vi "SynthApp.vi"(0 "Choose Directory":path, 1 "Show SF?":bool=TRUE, 2 "Show Sum?":bool, 3 "Save Center\nElem?":bool, 5 "Auto Select All?":bool, 7 "Use Selected Files":bool, 9 "Trans Geometry (mm)":T1={"Transducer"=0, "Geo Focus"=12.0, "a (radius)"=3.0, "# of rings"=5, "kerf space "=0.1, "Center Freq"=12.0} {"Transducer" items=["6D 12R 40 MHz"=0, "10D 31R 20 MHz"=1, "10D 23R 20 MHz"=2, "6D 23R 40 MHz"=3, "4.5D 10.7R 40 MHz"=4, "9D 23.5R 20 MHz"=5, "9D 25.8R 20MHz"=6, "Enter"=99]}, 11 "Method":u16(ring)=4 items=["Normal", "GPU", "ABUT", "EXPAND", "CPU"], 12 "Save Data":bool, 13 "Type of Mean":T3=enum."Filter", 14 "Filter Prams":T4={"low cutoff"=5, "order"=51, "high cutoff"=65}) -> ()   [LabVIEW 2022 SP3]
uses:
  ViewData/-ReadEye/TypeDefs/TypeofMean.ctl
  -AnnularRoutines/TransGeometry.ctl
  -AnnularRoutines/ArrayGeometry.ctl
  -AnnularRoutines/AnnularArray.ctl
  <vilib>/Analysis/4window.llb/Chebyshev Window (DBL).vi
  -SynthApperture/FastArraySum.vi
  -SynthApperture/FastArraySumSGL.vi
  <vilib>/Analysis/NI_AALBase.lvlib
  <vilib>/Analysis/NI_AALPro.lvlib
  GPU_HK/LabVIEW Example/riversideSAFilter-X64.dll
panel:
  in  "offset dual (mm)":dbl=15.0
  in  "Special Two Way":bool
  in  "Nested Files?":bool
  in  "Save Tiff?":bool
  in  "index (row)":i32
  out "Waveform Graph":dbl[][](graph)
  in  "downfactor":i32=1
  in  "Xmt/Rcv":cluster{"XMIT":bool[], "RCV":bool[]}={"XMIT"=[TRUE, TRUE, TRUE, TRUE, TRUE], "RCV"=[TRUE, TRUE, TRUE, TRUE, TRUE]}
  out "Comment":string
  out "Recip Table":i16[][](array[numeric])
  in  "delay":sgl format="%_3f"
  out "annuli rad (mm)":dbl[](array[numeric])
  in  "Special Save":bool
  out "GPU time (ms)":u32
  out "nError":i32
  in  "Scale Voltage?":bool=TRUE
  out "time per\nimage (ms)":u32
  in  "One Way Receive":bool
  in  "Compression Parameters.% taper":sgl
  in  "Display Plots":bool=TRUE
  in  "Axis scaling":bool=TRUE
  in  "Compress":bool
  in  "Round to ROC?":bool=TRUE
  out "ROC (m)":dbl=0.012
  out "Current File":string
  in  "file ext":string="*1to1*"
  out "zone size mm":dbl format="%#_3g"
  in  "Normalize Voltages":bool
  in  "c (m/s)":i32=1485
  out "Raw Summation":dbl[][](graph)
  in  "F- zones":i16=41
  out "Focal zones m":sgl[](array[numeric])=[0.0085, 0.009, 0.0095, 0.01, 0.0105, 0.011, 0.0115, 0.012, 0.0125, 0.013, 0.0135, 0.014, 0.0145, 0.015]
  out "Synth Aperture":dbl[][](graph)
  in  "Listbox":i32[](listbox)
  # "Dynamic Receive"
  # "RCV"
  # "XMIT"
  # "Obsolete"
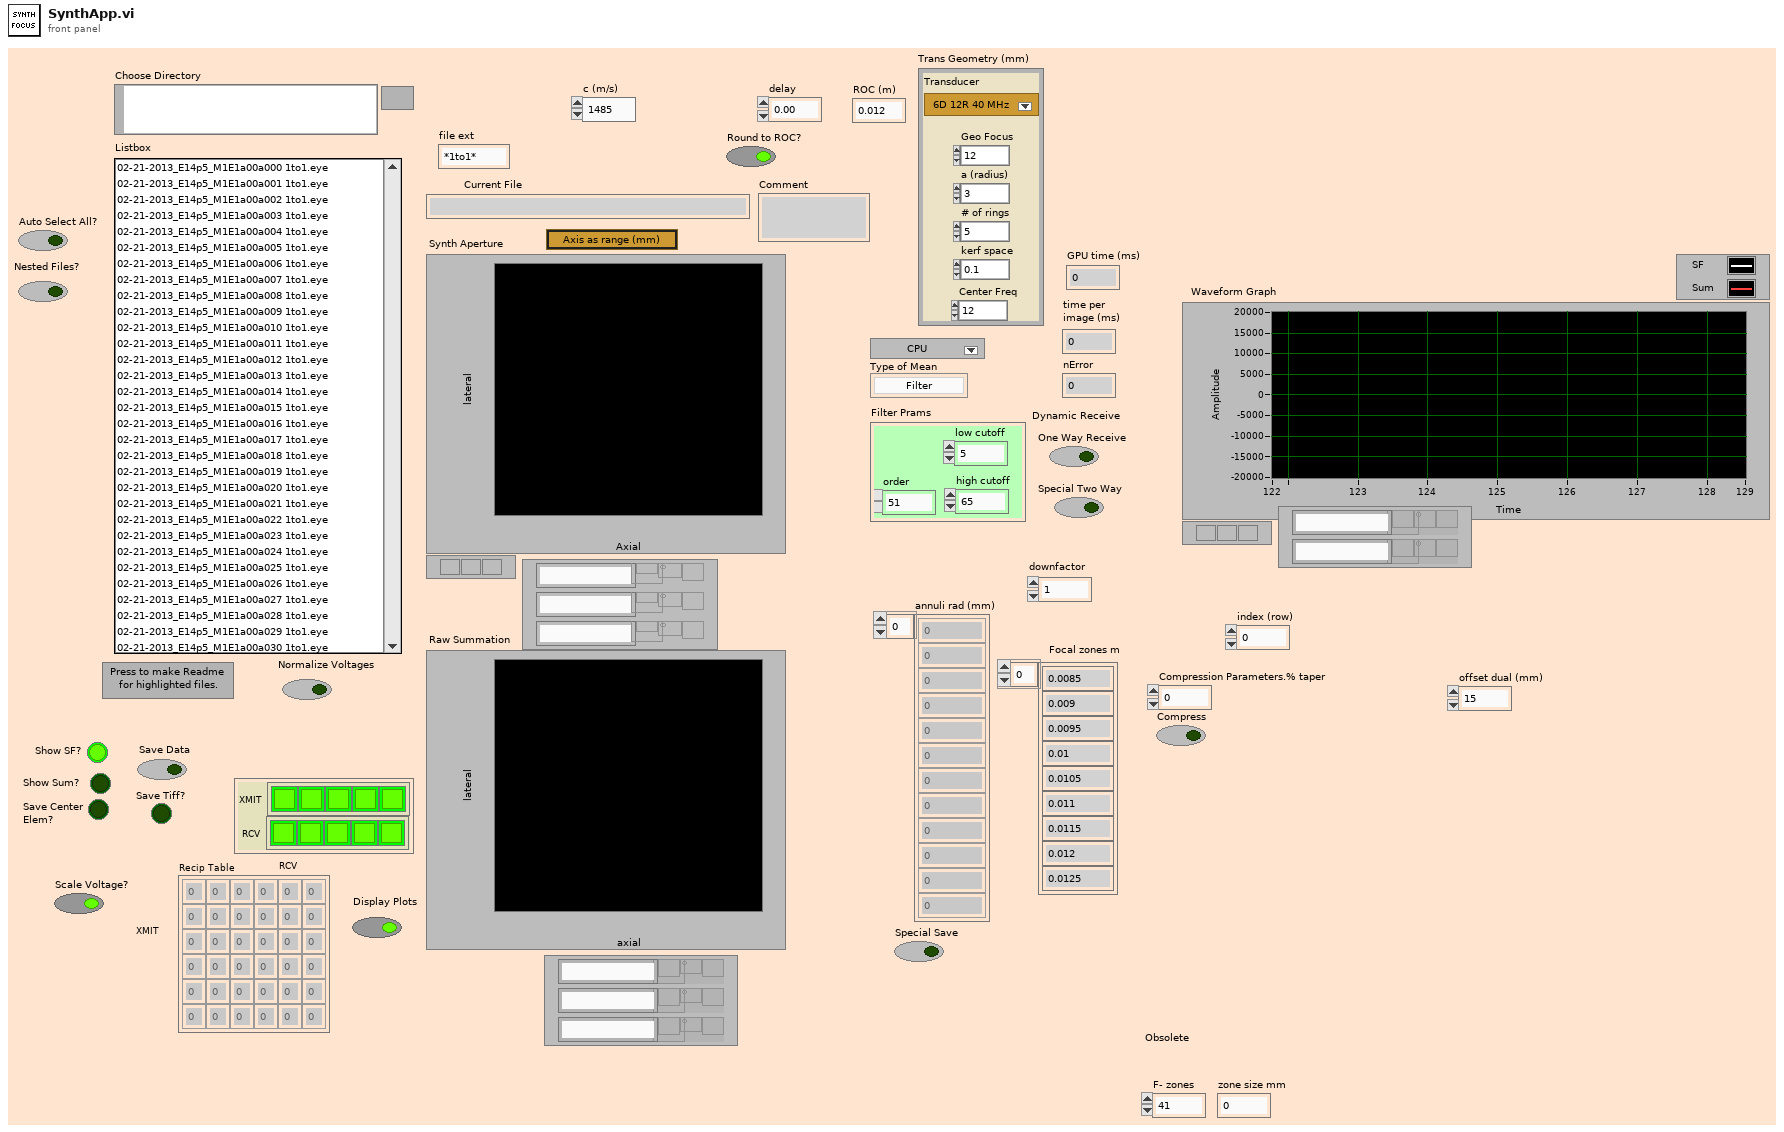
[diagram p1: front panel]
types:
  T1 = typedef "TransGeometry.ctl" = cluster{"Transducer":T2, "Geo Focus":dbl, "a (radius)":dbl, "# of rings":i32, "kerf space ":dbl, "Center Freq":dbl}
  T2 = typedef "ArrayGeometry.ctl" = u16
  T3 = typedef "TypeofMean.ctl" = enum16{"Mean from lines", "Mean just lines", "Poly Mean", "No mean", "Filter"}
  T4 = cluster{"low cutoff":i32, "order":i32, "high cutoff":i32}
  T5 = typedef "AnnularArray.ctl" = cluster{"Synth Foc?":bool, "Focal Zones":i16, "Switch T/R":i16, "Trans Geometry (mm)":T1, "Sub Ap Excite?":bool, "Full Array Scan?":bool, "Xmt/Rcv":cluster{"XMIT":bool[], "RCV":bool[]}, "PulseSpacing (us)":sgl, "Xmit Ring":i32, "XMIT CHS":u8, "RCV CHS":u8, "GPU?":bool, "Save TIFF?":bool, "downfactor":i32, "RCV 1CH":u16}
  T6 = cluster{"txPos":i32[], "rxPos":i32[], "Weights":i16[], "Ones":i16[]}
  T7 = typedef "Header.ctl" = cluster{"header info":cluster{"Header":string, "Head length":i16}, "A/D info":cluster{"# rf points per line":u16, "# lines per scan":u16, "sample rate MHz":u16, "# A/D bits":i16, "# bytes per A/D":u16, "TGC Flag":u16, "A/D Type":string}, "Tranducer Info":cluster{"bandwidth":sgl, "center freq":sgl, "start freq":sgl, "ID":i32}, "Scan Info":cluster{"delay":sgl, "pivot distance":sgl, "sector scan angle":sgl, "operator":string, "Scan Mode":string, "location":string}, "Time/Date Info":cluster{"date":string, "time":string}, "RF Info":cluster{"RF file name":string, "RF file att":string, "RF cal file name":string, "RF cal file att":string}, "Patient Info":cluster{"ID":string, "extended ID":string, "age":u16, "sex":string, "previously\nscanned":string, "PSA":sgl, "LOS":u8, "Ethnicty 2":u8, "Race":u8}, "Tissue Type":cluster{"organ":i16, "disease type":i16, "disease location":i16, "IQ_pts":u16, "RcvBuffer":u8, "RcvFrame":u16, "IQBuff":u8, "IQFrame":u16, "IQPage":u8}, "Votage scaling":cluster{"Digitizer (dB)":sgl, "Gain (dB)":sgl, "Atten (dB)":sgl}, "Comment":string, "Misc Info":cluster{"avg num":u16, "c speed":i16, "Div By or SF zones":i16, "XMIT CHS":u8, "RCV CHS":u8, "Xmit angle":sgl}, "Therapy Parameters":cluster{"Theraputic Freq (MHz)":sgl, "Time on (s)":sgl, "Therapy amplitude (mV)":sgl, "Lines Before":u16, "Lines After":u16}, "Scan Settings":cluster{"Energy (uJ or V)":u8, "Damp (Ohm) or Fc":u8, "HP Filt (KHz)":u8, "LP Filt (MHz)":u8, "Gain (db)":u8, "prf (kHz)":sgl, "Distance between\nscan lines (um)":u16, "Distance between\nscan planes (um)":u16, "Scan line gap (um)":sgl, "Scan plane gap (um)":sgl}, "Compression Parameters":cluster{"F1 (MHz)":sgl, "F2 (MHz)":sgl, "% taper":sgl, "duration":sgl}, "Patient Info Xtra":cluster{"First Name":string, "Last Name":string, "Notes":string}, "ROI Box":u16[]}
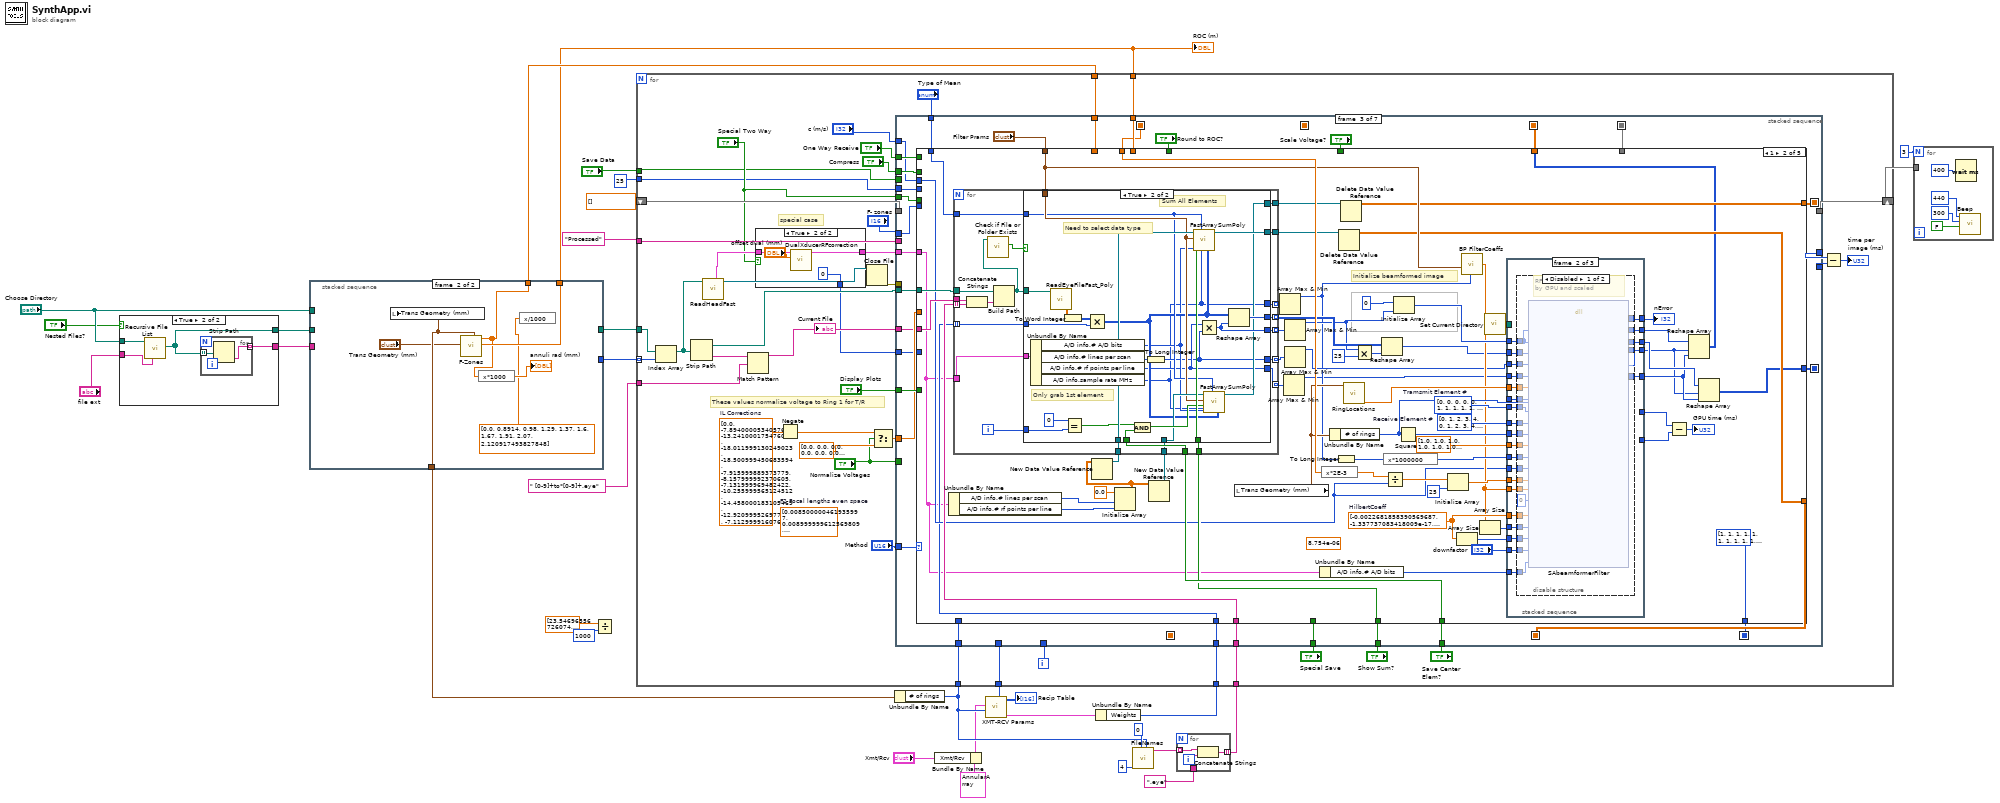
[diagram p0: block diagram]
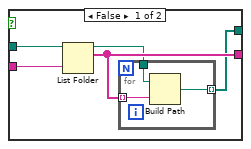
[diagram p2: hidden frame]
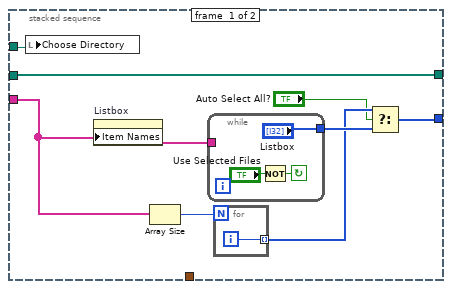
[diagram p3: hidden frame]
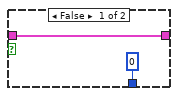
[diagram p4: hidden frame]
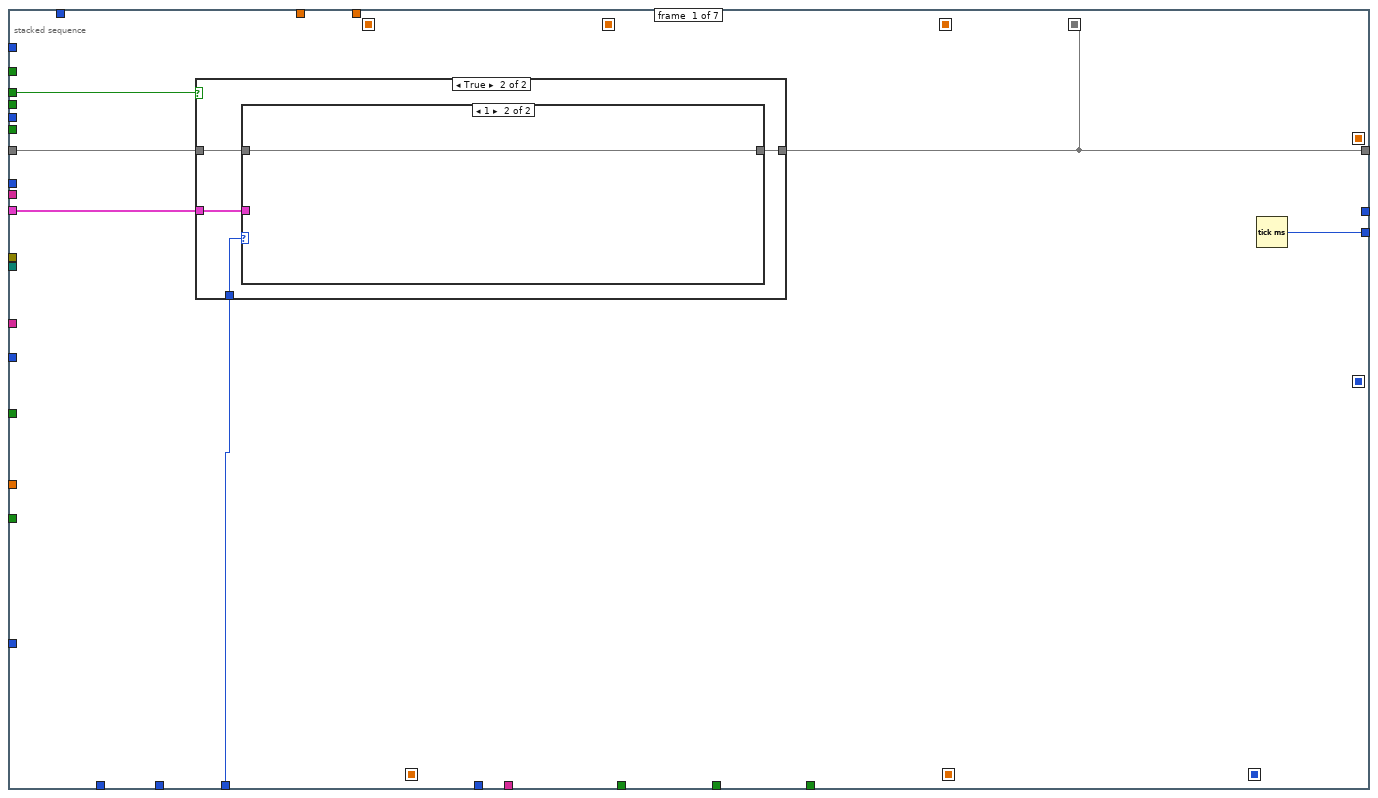
[diagram p5: hidden frame]
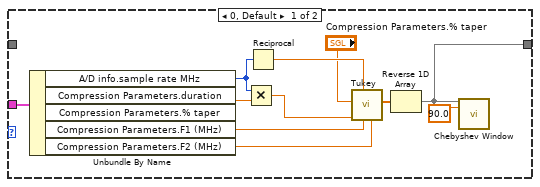
[diagram p7: hidden frame]
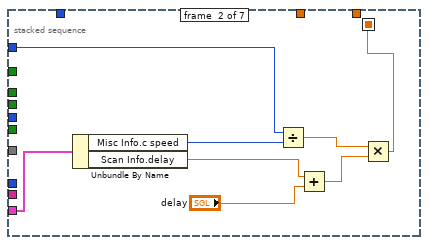
[diagram p8: hidden frame]
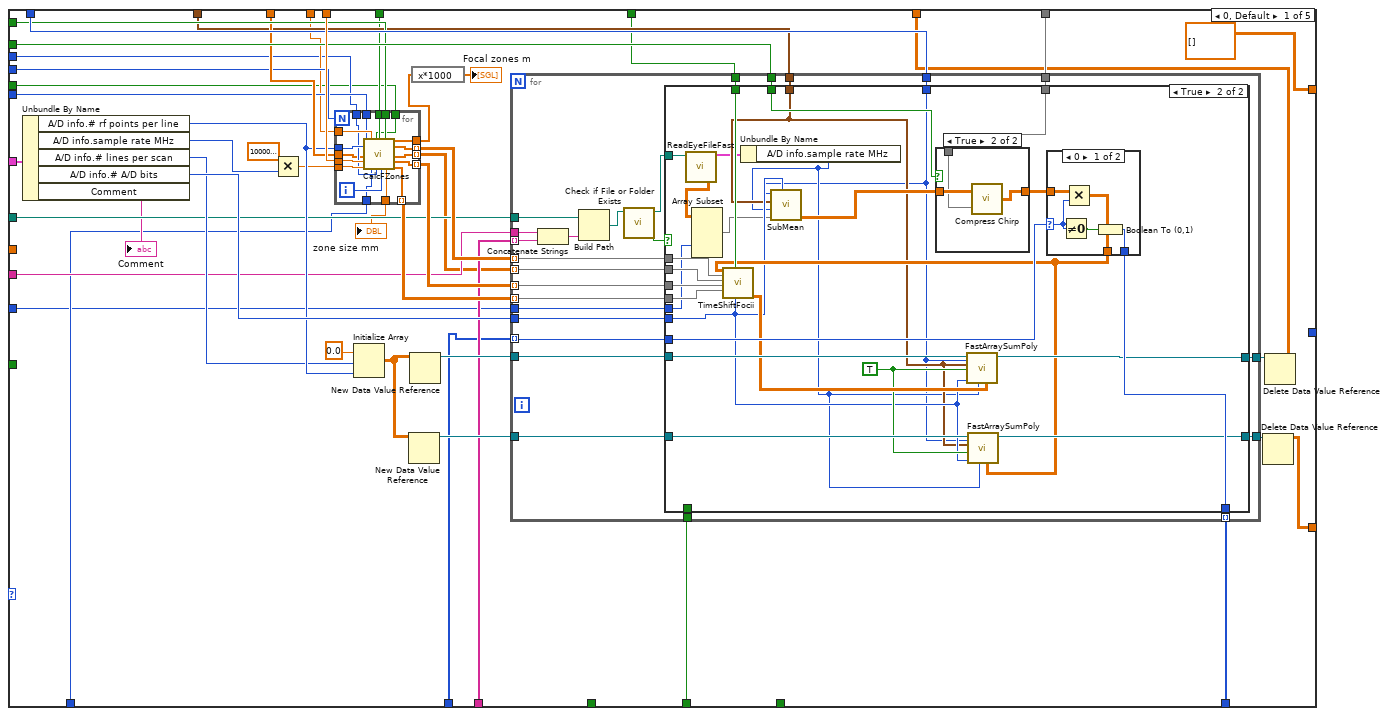
[diagram p9: hidden frame]
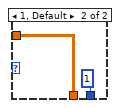
[diagram p11: hidden frame]
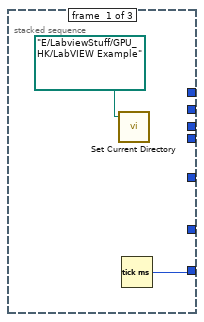
[diagram p13: hidden frame]
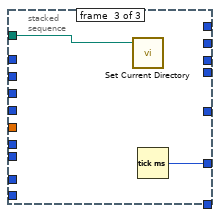
[diagram p15: hidden frame]
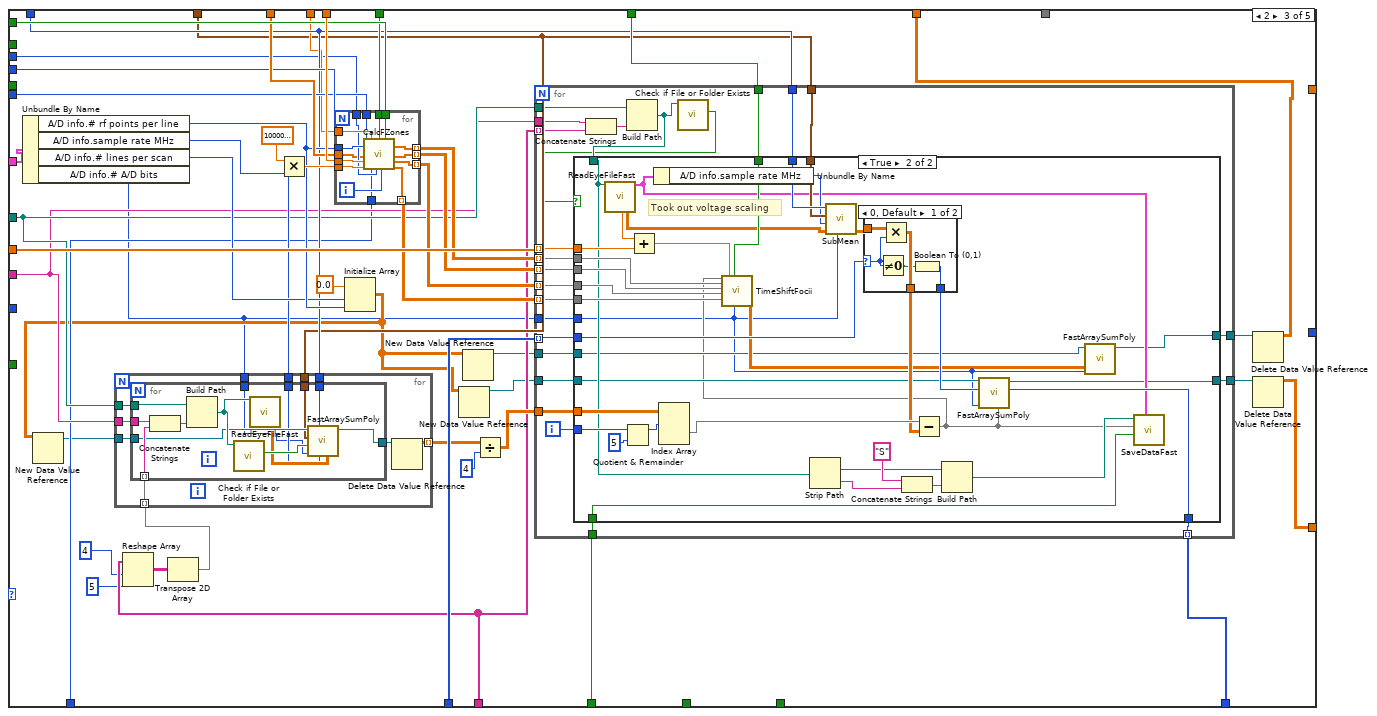
[diagram p17: hidden frame]
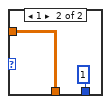
[diagram p19: hidden frame]
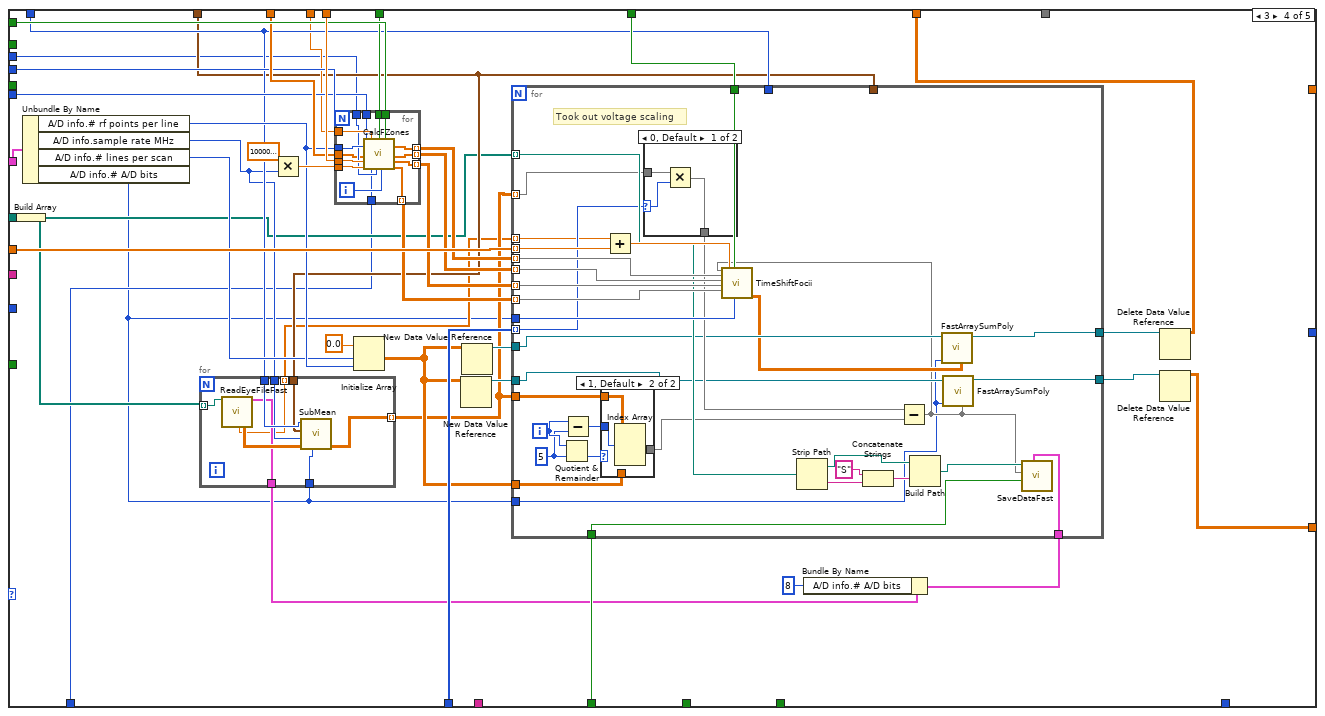
[diagram p20: hidden frame]
diagram:
  n1 = case shown="True" "Nested Files?" {
    tunnel: "file ext" -> [w37 w43]
    tunnel: "Choose Directory" -> [w36 w44]
    tunnel: [w35 w41] -> w12
    tunnel: [w33 w42] -> w10
    frame False {
      n2 = List Folder(path=w36, pattern=w37) -> (path out=w34:path, filenames=w35:string[])  [unwired: 1 in, 3 out]
      n3 = for {
        tunnel: w35 -> [w40] mode=indexing
        tunnel: w34 -> [w39]
        tunnel: [w38] -> w33 mode=indexing
        n4 = Build Path(base path=w39, name or relative path=w40) -> (appended path=w38:path)
      }
    }
    frame True {
      n5 = call <vilib>:"Recursive File List.vi"("pattern"=w43, "Folder Path"=w44) -> ("All Files in Dir"=w42:path[])  [unwired: 5 in, 4 out]
      n6 = for {
        tunnel: w42 -> [w46] mode=indexing
        tunnel: [w45] -> w41 mode=indexing
        n7 = Strip Path(path=w46) -> (name=w45:string)  [unwired: 1 out]
      }
    }
  }
  n8 = stacked-sequence {
    tunnel: "Choose Directory" -> [w54 _]
    tunnel: [w48 _] -> w32
    tunnel: [w47 _] -> w31
    tunnel: [_ w61] -> w29
    tunnel: [_ w64] -> w28
    tunnel: [_ w60] -> w22
    tunnel: w12 -> [w51 _]
    tunnel: w10 -> [w47 _]
    frame #0 {
      n9 = local write "Choose Directory"(w54) -> ()
      n10 = property on="Listbox" class="LstBox (strict)"("Item Names"=w51) -> ()  [unwired: 2 in, 2 out]
      n11 = Array Size(array=w51) -> (size(s)=w50:i32)
      n12 = while {
        tunnel: ["Listbox"] -> w53
        tunnel: w51 -> [_]
        stop <- w58 continue-if-true
        n13 = Not(x="Use Selected Files") -> (.not. x?=w58:bool)
      }
      n14 = for {
        N: w50 -> [_]
        tunnel: [w55] -> w52 mode=indexing
        i -> [w55]
      }
      n15 = Select(t=w52, s="Auto Select All?", f=w53) -> (s? t:f=w48:i32[])
    }
    frame #1 {
      n16 = call "F-Zones.vi"("Trans Geometry (mm)"="Trans Geometry (mm)") -> ("ROC (m)"=w64:dbl, "annuli rad (m)"=w61:dbl[], "Trans Geometry (mm) out"=w60:T1)  [unwired: 7 in, 1 out]
      n17 = local write "Trans Geometry (mm)"(w60) -> ()
      n18 = expression code="x*1000"(w61) -> (→"annuli rad (mm)":dbl[])
      n19 = expression code="x/1000"(dbl[] [0.0, 0.8914, 0.98, 1.29, 1.37, 1.6, 1.67, 1.91, 2.07, 2.120917493827848] ("annuli rad (mm)")) -> ()  [unwired: 1 out]
    }
  }
  "ROC (m)" <- w28
  n20 = Divide(x=dbl[] [23.54696556726074, 24.765259567260742, 25.794364567260743, 26.782632067260742, 27.77980956726074, 28.724764567260742, 29.665759567260743] ("Wire Locations mm"), y=1000) -> ()  [unwired: 1 out]
  n21 = Unbundle By Name(w22) -> ("# of rings"=w8:i32)
  n22 = Bundle By Name(cluster=T5 {"Synth Foc?"=TRUE, "Focal Zones"=41, "Switch T/R"=1, "Trans Geometry (mm)"={"Transducer"=0, "Geo Focus"=12.0, "a (radius)"=3.0, "# of rings"=5, "kerf space "=0.1, "Center Freq"=40.0}, "Sub Ap Excite?"=FALSE, "Full Array Scan?"=FALSE, "Xmt/Rcv"={"XMIT"=[TRUE, TRUE, TRUE, TRUE, TRUE], "RCV"=[TRUE, TRUE, TRUE, TRUE, TRUE]}, "PulseSpacing (us)"=0.0, "Xmit Ring"=0, "XMIT CHS"=5, "RCV CHS"=5, "GPU?"=TRUE, "Save TIFF?"=FALSE, "downfactor"=1, "RCV 1CH"=0} ("Ann Array Params"), "Xmt/Rcv"="Xmt/Rcv") -> (w5:T5)
  n23 = call "XMT-RCV Params.vi"("Dig Channels"=w8, "Ann Array Params"=w5) -> ("GPU ordering"=w2:T6, "Recip Table"=→"Recip Table":i16[][], "virtual T/R count"=w11:i16)  [unwired: 4 in, 3 out]
  n24 = Unbundle By Name(w2) -> ("Weights"=w1:i16[])
  n25 = call "FileNames.vi"("# Elements"=w8, "Digits"=0, "Dig Config"=4) -> ("All files"=w19:string[])  [unwired: 6 in, 2 out]
  n26 = for {
    tunnel: w19 -> [w67] mode=indexing
    tunnel: ".eye" -> [w66]
    tunnel: [w65] -> w17 mode=indexing
    n27 = Concatenate Strings(w67, w66) -> (w65:string)
  }
  n28 = for {
    tunnel: "Save Data" -> [w71]
    tunnel: "Processed" -> [w108]
    tunnel: w32 -> [w107] mode=indexing
    tunnel: w31 -> [w82]
    tunnel: w29 -> [w106]
    tunnel: w28 -> [w105]
    shift-right: [w102] -> w16
    shift-left: dbl[] [] ("FFT {X}") -> [w103]
    tunnel: 25 -> [w72]
    tunnel: " [0-9]+to*[0-9]+.eye" ("string") -> [w88]
    tunnel: w17 -> [w86]
    tunnel: w8 -> [w85]
    tunnel: w11 -> [w83]
    tunnel: w1 -> [w78]
    i -> [w104]
    (unwired) sgl[] [0.0085, 0.009, 0.0095, 0.01, 0.0105, 0.011, 0.0115, 0.012, 0.0125, 0.013, 0.0135, 0.014, 0.0145, 0.015]  # F2 Focal lengths even space
    w109 = sgl[] [0.0, -7.894, -13.241, -18.012, -18.501, -7.916, -8.158, -7.132, -10.256, -14.458, -12.921, -7.113, -8.934, -6.912, -8.33, -18.133, -10.341, -6.825, -9.709, -9.301, -18.345, -14.547, -8.321, -9.392, -7.948]  # IL Corrections
    # "special case"
    # "These values normalize voltage to Ring 1 for T/R"
    n29 = Index Array(array=w82, index=w107) -> (element=w80:path)
    n30 = Strip Path(path=w80) -> (stripped path=w79:path, name=w81:string)
    n31 = call "ReadHeadFast.vi"("new file path"=w80) -> ("refnum out"=w75:refnum<file>, "Header In"=w77:T7)  [unwired: 7 in, 2 out]
    n32 = Match Pattern(string=w81, regular expression=w88) -> (before substring=w87:string)  [unwired: 1 in, 3 out]
    "Current File" <- w87
    n33 = case shown="True" "Special Two Way" {
      tunnel: w77 -> [w112 w116]
      tunnel: [w112 w115] -> w76
      tunnel: [0 ("pts to cut") 0 ("pts to cut")] -> w74
      frame False {
      }
      frame True {
        n34 = call "DualXducerRFcorrection.vi"("distance correction mm"="offset dual (mm)", "Header In"=w116) -> ("Header modified"=w115:T7)  [unwired: 5 in, 1 out]
      }
    }
    n35 = Negate(x=w109) -> (-x=w98:sgl[])
    n36 = Close File(refnum=w75) -> (error out=w90:errorcluster)  [unwired: 1 in, 1 out]
    n37 = Select(t=w98, s="Normalize Voltages", f=sgl[] [0.0, 0.0, 0.0, 0.0, 0.0, 0.0, 0.0, 0.0, 0.0, 0.0, 0.0, 0.0, 0.0, 0.0, 0.0, 0.0, 0.0, 0.0, 0.0, 0.0, 0.0, 0.0, 0.0, 0.0, 0.0]) -> (s? t:f=w99:sgl[])
    n38 = stacked-sequence {
      seq-local: [_ _ w177 _ _ _ _] -> [_ _ _ w834 _ _ w963]
      seq-local: [_ _ w172 _ _ _ _] -> [_ _ _ w833 _ _ w962]
      seq-local: [_ _ _ w861 _ _ _] -> [_ _ _ _ _ _ w979]
      seq-local: [w118 _ _ _ _ _ _] -> [_ _ w174 _ _ _ _]
      seq-local: [_ w142 _ _ _ _ _] -> [_ _ w159 _ w901 _ w974]
      seq-local: [_ _ w157 _ _ _ _] -> [_ _ _ w841 _ _ _]
      seq-local: [_ _ _ w835 _ _ _] -> [_ _ _ _ _ _ w972]
      seq-local: [_ _ w151 _ _ _ _] -> [_ _ _ _ _ _ w965]
      seq-local: [_ _ w150 _ _ _ _] -> [_ _ _ _ _ _ w961]
      tunnel: w76 -> [w121 w147 w179 w840 w907 _ w980]
      tunnel: "F- zones" -> [_ _ w178 _ _ _ w978]
      tunnel: w99 -> [_ _ w168 _ _ _ _]
      tunnel: w79 -> [_ _ w173 _ _ w951 w966]
      tunnel: w71 -> [_ _ _ _ _ w953 w975]
      tunnel: "Normalize Voltages" -> [_ _ _ _ _ _ w977]
      tunnel: w108 -> [_ _ _ _ _ w952 w976]
      tunnel: w106 -> [_ _ w167 _ w902 _ _]
      tunnel: w105 -> [_ _ w176 _ w903 _ _]
      tunnel: w104 -> [w122 _ _ _ _ _ _]
      tunnel: w103 -> [w120 _ _ _ _ _ _]
      tunnel: [w118 _ _ _ _ _ _] -> w102
      tunnel: "Compress" -> [w119 _ w175 _ _ _ _]
      tunnel: "Display Plots" -> [_ _ w169 w851 w906 _ _]
      tunnel: "Type of Mean" -> [_ _ w171 _ _ _ _]
      tunnel: "One Way Receive" -> [_ _ w170 _ w905 _ _]
      tunnel: [w117 _ _ _ _ _ _] -> w94
      tunnel: [_ _ _ w850 _ _ _] -> w95
      tunnel: w72 -> [_ _ w166 _ _ _ _]
      tunnel: "Method" -> [_ _ w165 w849 w904 _ _]
      tunnel: w78 -> [_ _ w161 _ _ _ _]
      tunnel: "Special Save" -> [_ _ w160 _ _ _ _]
      tunnel: "c (m/s)" -> [_ w144 w158 _ w900 _ w973]
      tunnel: w90 -> [_ _ _ _ _ _ _]
      tunnel: "Show Sum?" -> [_ _ w156 _ _ _ w968]
      tunnel: w87 -> [_ _ w155 _ _ _ w967]
      tunnel: w86 -> [_ _ w154 _ _ _ _]
      tunnel: w85 -> [_ _ w153 _ _ _ _]
      tunnel: "Save Center\nElem?" -> [_ _ w152 _ _ _ w964]
      tunnel: w83 -> [_ _ _ _ _ _ w960]
      tunnel: "Special Two Way" -> [_ _ w149 _ _ _ _]
      tunnel: w74 -> [_ _ w148 _ _ _ _]
      frame #0 {
        n39 = case shown="True" w119 {
          tunnel: w122 -> [_ w127]
          tunnel: w121 -> [_ w126]
          tunnel: w120 -> [w123 w125]
          tunnel: [w123 w124] -> w118
          frame False {
          }
          frame True {
            n40 = case shown="1" w127 {
              tunnel: w126 -> [w133 _]
              tunnel: w125 -> [_ w139]
              tunnel: [w129 w139] -> w124
              frame 0, Default {
                n41 = Unbundle By Name(w133) -> ("A/D info.sample rate MHz"=w131:u16, "Compression Parameters.duration"=w135:sgl, "Compression Parameters.F1 (MHz)"=w137:sgl, "Compression Parameters.F2 (MHz)"=w138:sgl)  [unwired: 1 out]
                n42 = Multiply(x=w131, y=w135) -> (x*y=w134:sgl)
                n43 = Reciprocal(x=w131) -> (1/x=w136:dbl)
                n44 = call "Tukey.vi"("f2 (MHz)"=w138, "f1 (MHz)"=w137, "Samp Rate (mics)"=w136, "Pts"=w134, "Tukey"="Compression Parameters.% taper") -> ("Tukey Chirp"=w132:dbl[])  [unwired: 2 in, 4 out]
                n45 = Reverse 1D Array(array=w132) -> (reversed array=w129:dbl[])
                n46 = call-poly <vilib>:"Chebyshev Window.vi"("lobe ratio (dB)"=90.0, "X"=w129) -> ()  [unwired: 10 out]
              }
              frame 1 {
              }
            }
          }
        }
        n47 = Tick Count (ms)() -> (millisecond timer value=w117:u32)
      }
      frame #1 {
        n48 = Unbundle By Name(w147) -> ("Misc Info.c speed"=w146:i16, "Scan Info.delay"=w141:sgl)
        n49 = Divide(x=w144, y=w146) -> (x/y=w145:dbl)
        n50 = Add(x=w141, y="delay") -> (x+y=w140:sgl)
        n51 = Multiply(x=w145, y=w140) -> (x*y=w142:dbl)
      }
      frame #2 {
        n52 = case shown="1" w165 {
          tunnel: w179 -> [w189 w313 w487 w644 w743]
          tunnel: w178 -> [w210 _ w508 w656 _]
          tunnel: [w204 w310 w483 w637 w755] -> w177
          tunnel: w176 -> [w223 _ w520 w668 w768]
          tunnel: w175 -> [w222 _ _ _ w767]
          tunnel: w174 -> [w221 _ _ _ w766]
          tunnel: w173 -> [w193 w356 w495 w652 w746]
          tunnel: [w200 w338 w480 w636 w751] -> w172
          tunnel: w171 -> [w220 w333 w501 w650 w765]
          tunnel: w170 -> [w219 _ w519 w667 w764]
          tunnel: w169 -> [_ _ _ _ _]
          tunnel: w168 -> [_ _ w518 w666 _]
          tunnel: w167 -> [w217 _ w515 w663 w763]
          tunnel: w166 -> [w216 _ w514 w662 _]
          tunnel: "Filter Prams" -> [w209 w339 w498 w648 w759]
          tunnel: "Scale Voltage?" -> [w208 _ w506 w655 w758]
          tunnel: "Round to ROC?" -> [w207 _ w505 w654 _]
          tunnel: w161 -> [w185 w322 w504 w653 w740]
          tunnel: w160 -> [_ _ w500 w651 _]
          tunnel: w158 -> [w196 w324 w496 w646 w748]
          tunnel: w159 -> [w199 w357 w499 w649 w750]
          tunnel: [w198 i32[] [1, 1, 1, 1, 1, 1, 1, 1, 1, 1, 1, 1, 1, 1, 1, 1, 1, 1, 1, 1, 1, 1, 1, 1, 1] w488 _ w749] -> w157
          tunnel: w156 -> [w194 w325 _ _ w747]
          tunnel: w155 -> [w192 w355 w494 _ w745]
          tunnel: w154 -> [w191 w354 w493 _ w744]
          tunnel: w153 -> [w188 _ w486 w643 _]
          tunnel: w152 -> [_ w326 _ _ _]
          tunnel: [dbl[][] [] w328 _ _ dbl[][] []] -> w151
          tunnel: [_ w309 _ _ _] -> w150
          tunnel: w149 -> [w184 _ _ _ w739]
          tunnel: w148 -> [w183 _ _ _ w738]
          frame 0, Default {
            n53 = Unbundle By Name(w189) -> ("A/D info.# rf points per line"=w212:u16, "A/D info.sample rate MHz"=w213:u16, "A/D info.# lines per scan"=w211:u16, "A/D info.# A/D bits"=w224:i16, "Comment"=→"Comment":string)
            n54 = Multiply(x=1000000.0, y=w213) -> (x*y=w180:dbl)
            n55 = for {
              N: w216 -> [_]
              tunnel: w199 -> [w243]
              tunnel: w210 -> [w242]
              tunnel: w212 -> [w241]
              tunnel: w180 -> [w240]
              tunnel: [w239] -> w197
              tunnel: w223 -> [w238]
              tunnel: w196 -> [w237]
              tunnel: w207 -> [w236]
              tunnel: w219 -> [w235]
              tunnel: [w234] -> w218 mode=indexing
              tunnel: [w233] -> w186 mode=indexing
              tunnel: w217 -> [w232]
              tunnel: [w230] -> w181
              tunnel: [w229] -> w215 mode=indexing
              tunnel: [w228] -> w214 mode=indexing
              tunnel: w188 -> [w227]
              tunnel: w184 -> [w226]
              i -> [w231]
              n56 = call "CalcFZones.vi"("F- zones"=w242, "# rf points per line"=w241, "Radii (m)"=w232, "ROC (m)"=w238, "Sampling Rate"=w240, "delay (mm)"=w243, "# Elements"=w227, "Dual mode"=w226, "c (m/s)"=w237, "Round to ROC?"=w236, "File index number"=w231, "One Way Receive"=w235) -> ("zone size mm"=w230:dbl, "FZones (m)"=w239:dbl[], "ZoneStart"=w234:sgl[], "ZoneShift"=w233:sgl[], "ZoneLength"=w228:sgl[], "IndexVals"=w229:sgl[])  [unwired: 2 in]
            }
            "zone size mm" <- w181
            n57 = Initialize Array(0.0, w211, w212) -> (w203:dbl[][])
            n58 = New Data Value Reference(data value=w203) -> (data value reference=w202:refnum<data-value>)  [unwired: 1 in, 1 out]
            n59 = New Data Value Reference(data value=w203) -> (data value reference=w206:refnum<data-value>)  [unwired: 1 in, 1 out]
            n60 = expression code="x*1000"(w197) -> (→"Focal zones m":dbl[])
            n61 = for {
              tunnel: w224 -> [w265]
              tunnel: w221 -> [w267]
              tunnel: w222 -> [w268]
              tunnel: w209 -> [w256]
              tunnel: w220 -> [w266]
              tunnel: w185 -> [w253] mode=indexing
              tunnel: w218 -> [w254] mode=indexing
              tunnel: w186 -> [w261] mode=indexing
              tunnel: w208 -> [w264]
              tunnel: w215 -> [w263] mode=indexing
              tunnel: w214 -> [w262] mode=indexing
              tunnel: w206 -> [w260]
              tunnel: [w259] -> w205
              tunnel: w202 -> [w258]
              tunnel: [w257] -> w201
              tunnel: [w255] -> w198 mode=indexing
              tunnel: w194 -> [w252]
              tunnel: w193 -> [w251]
              tunnel: w192 -> [w249]
              tunnel: w191 -> [w248] mode=indexing
              tunnel: w183 -> [w244]
              n62 = Concatenate Strings(w249, w248) -> (w247:string)
              n63 = Build Path(base path=w251, name or relative path=w247) -> (appended path=w245:path)
              n64 = call <vilib>:"Check if File or Folder Exists.vi"("path"=w245) -> ("file or folder exists?"=w246:bool, "dup path"=w250:path)  [unwired: 8 in, 1 out]
              n65 = case shown="True" w246 {
                tunnel: w268 -> [_ w297]
                tunnel: w267 -> [_ w296]
                tunnel: w250 -> [_ w295]
                tunnel: w266 -> [_ w275]
                tunnel: w265 -> [_ w278]
                tunnel: w264 -> [_ w293]
                tunnel: w263 -> [_ w292]
                tunnel: w262 -> [_ w291]
                tunnel: w261 -> [_ w290]
                tunnel: w260 -> [w270 w286]
                tunnel: [w270 w285] -> w259
                tunnel: w258 -> [w269 w283]
                tunnel: [w269 w282] -> w257
                tunnel: w256 -> [_ w277]
                tunnel: [_ w289] -> w255
                tunnel: w254 -> [_ w288]
                tunnel: w253 -> [_ w287]
                tunnel: w252 -> [_ _]
                tunnel: w244 -> [_ w271]
                frame False {
                }
                frame True {
                  w280 = TRUE ("Perform Sum?")
                  n66 = call "ReadEyeFileFast.vi"("new file path"=w295) -> ("2-D data array"=w273:sgl[][], "Header In"=w274:T7)  [unwired: 1 in, 16 out]
                  n67 = Array Subset(array=w273, index (col)=w271) -> (w272:sgl[][])  [unwired: 3 in]
                  n68 = Unbundle By Name(w274) -> ("A/D info.sample rate MHz"=w276:u16)
                  n69 = call "SubMean.vi"("Bit Depth"=w278, "Scan Data In"=w272, "Samp Rate (MHz)"=w276, "Filter Prams"=w277, "Type of Mean"=w275) -> ("Array"=w279:dbl[][])  [unwired: 1 in, 2 out]
                  n70 = case shown="True" w297 {
                    tunnel: [w305 w308] -> w294
                    tunnel: w279 -> [w305 w307]
                    tunnel: w296 -> [_ w306]
                    frame False {
                    }
                    frame True {
                      n71 = call "Compress Chirp.vi"("Chirp"=w306, "Array In"=w307) -> ("Array Out"=w308:dbl[][])
                    }
                  }
                  n72 = case shown="0" w287 {
                    selector: w287 -> [w298 _]
                    tunnel: w294 -> [w302 w304]
                    tunnel: [w301 w304] -> w281
                    tunnel: [w299 i16 1] -> w289
                    frame 0 {
                      n73 = Not Equal To 0?(x=w298) -> (x != 0?=w300:bool)
                      n74 = Multiply(x=w302, y=w298) -> (x*y=w301:dbl[][])
                      n75 = Boolean To (0,1)(Boolean=w300) -> (0, 1=w299:i16)
                    }
                    frame 1, Default {
                    }
                  }
                  n76 = call "TimeShiftFocii.vi"("Array data"=w281, "ZoneStart"=w288, "ZoneShift"=w290, "ZoneLength"=w291, "IndexVals"=w292, "Scale Voltage?"=w293, "A/D info.# A/D bits"=w278) -> ("Synth App Out"=w284:dbl[][])  [unwired: 12 in]
                  n77 = call-poly "FastArraySumPoly.vi"("2-D data array"=w284, "sample rate MHz"=w276, "Type of Mean"=w275, "Bit Depth"=w278, "Perform Sum?"=w280, "Filter Prams"=w277, "Data Value Reference in"=w286) -> ("Data Value Reference out"=w285:refnum<data-value>)  [unwired: 4 in]
                  n78 = call-poly "FastArraySumPoly.vi"("2-D data array"=w281, "sample rate MHz"=w276, "Type of Mean"=w275, "Bit Depth"=w278, "Perform Sum?"=w280, "Filter Prams"=w277, "Data Value Reference in"=w283) -> ("Data Value Reference out"=w282:refnum<data-value>)  [unwired: 4 in]
                }
              }
            }
            n79 = Delete Data Value Reference(data value reference=w201) -> (data value=w200:dbl[][])  [unwired: 1 in, 1 out]
            n80 = Delete Data Value Reference(data value reference=w205) -> (data value=w204:dbl[][])  [unwired: 1 in, 1 out]
          }
          frame 1 {
            w345 = sgl[] [-0.0022681858, -1.3377371e-17, -0.0041749156, 1.3026156e-17, -0.0068346895, -4.195826e-17, -0.010427003, -1.1244341e-16, -0.015182828, -3.725316e-17, -0.021423787, -1.1259981e-16, -0.029640518, -9.678795e-17, -0.040659484, -5.638797e-17, -0.05603469, 9.1425055e-18, -0.079112425, -9.958648e-17, -0.118650794, 1.000237e-18, -0.20691232, -6.3757414e-17, -0.6348398, 0.0, 0.6348398, 6.3757414e-17, 0.20691232, -1.000237e-18, 0.118650794, 9.958648e-17, 0.079112425, -9.1425055e-18, 0.05603469, 5.638797e-17, 0.040659484, 9.678795e-17, 0.029640518, 1.1259981e-16, 0.021423787, 3.725316e-17, 0.015182828, 1.1244341e-16, 0.010427003, 4.195826e-17, 0.0068346895, -1.3026156e-17, 0.0041749156, 1.3377371e-17, 0.0022681858]  # HilbertCoeff
            (unwired) 8.754e-06
            w346 = i32[] [0, 1, 2, 3, 4, 0, 1, 2, 3, 4, 0, 1, 2, 3, 4, 0, 1, 2, 3, 4, 0, 1, 2, 3, 4, 0, 1, 2, 3, 4, 0, 1, 2, 3, 4, 0, 1, 2, 3, 4, 0, 1, 2, 3, 4, 0, 1, 2, 3, 4]  # Receive Element #
            w347 = i32[] [0, 0, 0, 0, 0, 1, 1, 1, 1, 1, 2, 2, 2, 2, 2, 3, 3, 3, 3, 3, 4, 4, 4, 4, 4, 0, 0, 0, 0, 0, 1, 1, 1, 1, 1, 2, 2, 2, 2, 2, 3, 3, 3, 3, 3, 4, 4, 4, 4, 4]  # Tramsmit Element #
            # "Initialize beamformed image"
            n81 = Unbundle By Name(w313) -> ("A/D info.# lines per scan"=w327:u16, "A/D info.# rf points per line"=w334:u16)
            n82 = Initialize Array(0.0, w327, w334) -> (w331:dbl[][])
            n83 = New Data Value Reference(data value=w331) -> (data value reference=w336:refnum<data-value>)  [unwired: 1 in, 1 out]
            n84 = New Data Value Reference(data value=w331) -> (data value reference=w329:refnum<data-value>)  [unwired: 1 in, 1 out]
            n85 = for {
              tunnel: [w433] -> w332 mode=indexing
              tunnel: [w449] -> w364 mode=indexing
              tunnel: [w446] -> w368 mode=indexing
              tunnel: [w448] -> w340 mode=indexing
              tunnel: [w447] -> w349 mode=indexing
              tunnel: w356 -> [w444]
              tunnel: w355 -> [w442]
              tunnel: w354 -> [w443] mode=indexing
              tunnel: w333 -> [w432]
              tunnel: w339 -> [w434]
              tunnel: w325 -> [w441]
              tunnel: w336 -> [w440]
              tunnel: [w439] -> w335
              tunnel: [w435] -> w330
              tunnel: w329 -> [w436]
              tunnel: w326 -> [w438]
              tunnel: w322 -> [w431] mode=indexing
              tunnel: w313 -> [w428]
              i -> [w437]
              n86 = Concatenate Strings(w442, w443) -> (w445:string)
              n87 = Build Path(base path=w444, name or relative path=w445) -> (appended path=w430:path)
              n88 = call <vilib>:"Check if File or Folder Exists.vi"("path"=w430) -> ("file or folder exists?"=w429:bool)  [unwired: 8 in, 2 out]
              n89 = case shown="True" w429 {
                tunnel: [_ w456] -> w449
                tunnel: [_ w476] -> w448
                tunnel: [_ w475] -> w447
                tunnel: [_ w454] -> w446
                tunnel: w441 -> [_ w474]
                tunnel: w430 -> [_ w473]
                tunnel: w440 -> [w450 w472]
                tunnel: [w450 w471] -> w439
                tunnel: w438 -> [_ w470]
                tunnel: w437 -> [_ w467]
                tunnel: w436 -> [w451 w465]
                tunnel: [w451 w464] -> w435
                tunnel: w434 -> [_ w463]
                tunnel: [_ w452] -> w433
                tunnel: w432 -> [_ w462]
                tunnel: w431 -> [_ w461]
                tunnel: w428 -> [_ w458]
                frame False {
                }
                frame True {
                  # "Only grab 1st element"
                  # "Sum All Elements"
                  # "Need to select data type"
                  n90 = Unbundle By Name(w458) -> ("A/D info.# A/D bits"=w457:i16, "A/D info.# lines per scan"=w455:u16, "A/D info.# rf points per line"=w456:u16, "A/D info.sample rate MHz"=w452:u16)
                  n91 = call-poly "ReadEyeFileFast_Poly.vi"("new file path"=w473) -> ("2-D data array"=w460:sgl[][])  [unwired: 13 in, 5 out]
                  n92 = To Word Integer(number=w460) -> (16bit integer=w453:i16[][])
                  n93 = Equal?(x=0, y=w467) -> (x = y?=w469:bool)
                  n94 = Multiply(x=w453, y=w461) -> (x*y=w459:i16[][])
                  n95 = And(x=w469, y=w470) -> (x .and. y?=w466:bool)
                  n96 = To Long Integer(number=w455) -> (32bit integer=w454:i32)
                  n97 = call-poly "FastArraySumPoly.vi"("2-D data array"=w459, "sample rate MHz"=w452, "Type of Mean"=w462, "Bit Depth"=w457, "Perform Sum?"=w474, "Filter Prams"=w463, "Data Value Reference in"=w472) -> ("Data Value Reference out"=w471:refnum<data-value>)  [unwired: 4 in]
                  n98 = Multiply(x=w456, y=w454) -> (x*y=w475:i32)
                  n99 = call-poly "FastArraySumPoly.vi"("2-D data array"=w459, "sample rate MHz"=w452, "Type of Mean"=w462, "Bit Depth"=w457, "Perform Sum?"=w466, "Filter Prams"=w463, "Data Value Reference in"=w465) -> ("Data Value Reference out"=w464:refnum<data-value>)  [unwired: 4 in]
                  n100 = Reshape Array(w459, w475) -> (w476:i16[])
                }
              }
            }
            n101 = local read "Trans Geometry (mm)"() -> (w353:T1)
            n102 = Array Max & Min(array=w332) -> (max value=w316:u16)  [unwired: 3 out]
            n103 = Array Max & Min(array=w364) -> (max value=w315:u16)  [unwired: 3 out]
            n104 = Array Max & Min(array=w349) -> (max value=w317:i32)  [unwired: 3 out]
            n105 = Array Max & Min(array=w368) -> (max value=w318:i32)  [unwired: 3 out]
            n106 = Unbundle By Name(w313) -> ("A/D info.# A/D bits"=w312:i16)
            n107 = expression code="x*2E-3"(w357) -> (w371:dbl)
            n108 = Unbundle By Name(w353) -> ("# of rings"=w351:i32)
            n109 = To Long Integer(number=w316) -> (32bit integer=w323:i32)
            n110 = Delete Data Value Reference(data value reference=w335) -> (data value=w338:dbl[][])  [unwired: 1 in, 1 out]
            n111 = Delete Data Value Reference(data value reference=w330) -> (data value=w328:dbl[][])  [unwired: 1 in, 1 out]
            n112 = call "RingLocations.vi"("Trans Geometry (mm)"=w353) -> ("GPU Geometry"=w343:dbl[])  [unwired: 9 in, 1 out]
            n113 = Multiply(x=w317, y=25) -> (x*y=w350:i32)
            n114 = Reshape Array(w340, w350) -> (w314:i16[])
            n115 = expression code="x*1000000"(w323) -> (w365:i32)
            n116 = Divide(x=w371, y=w324) -> (x/y=w358:dbl)
            n117 = Initialize Array(i16 0 ("element"), w317) -> (w370:i16[])
            n118 = Square(x=w351) -> (x^2=w352:i32)
            n119 = Initialize Array(w358, 25 ("Number of Tx/Rx pair")) -> (w366:dbl[])
            n120 = Array Size(array=w345) -> (size(s)=w311:i32)
            n121 = call "BP FilterCoeffs.vi"("sample rate MHz"=w316, "Filter Prams"=w339) -> ("FIR Windowed Coefficients"=w341:dbl[])  [unwired: 4 in]
            n122 = Array Size(array=w341) -> (size(s)=w344:i32)
            n123 = call "Set Current Directory.vi"() -> ("Get Directory"=w359:path)  [unwired: 5 in]
            n124 = stacked-sequence {
              tunnel: w370 -> [_ w390 _]
              tunnel: [_ w388 _] -> w369
              tunnel: w318 -> [_ w399 _]
              tunnel: w351 -> [_ w396 _]
              tunnel: w352 -> [_ w395 _]
              tunnel: sgl[] [1.0, 1.0, 1.0, 1.0, 1.0, 1.0, 1.0, 1.0, 1.0, 1.0, 1.0, 1.0, 1.0, 1.0, 1.0, 1.0, 1.0, 1.0, 1.0, 1.0, 1.0, 1.0, 1.0, 1.0, 1.0, 1.0, 1.0, 1.0, 1.0, 1.0, 1.0, 1.0, 1.0, 1.0, 1.0, 1.0, 1.0, 1.0, 1.0, 1.0, 1.0, 1.0, 1.0, 1.0, 1.0, 1.0, 1.0, 1.0, 1.0, 1.0] ("weighting") -> [_ w394 _]
              tunnel: w366 -> [_ w391 _]
              tunnel: w365 -> [_ w393 _]
              tunnel: w314 -> [_ w400 _]
              tunnel: w315 -> [_ w398 _]
              tunnel: w343 -> [_ w397 _]
              tunnel: w324 -> [_ w392 _]
              tunnel: [_ w387 _] -> w363
              tunnel: [_ _ w427] -> w361
              tunnel: [w376 _ _] -> w360
              tunnel: w359 -> [_ _ w426]
              tunnel: w341 -> [_ w389 _]
              tunnel: [_ w386 _] -> w321
              tunnel: w345 -> [_ w385 _]
              tunnel: w347 -> [_ w384 _]
              tunnel: w346 -> [_ w383 _]
              tunnel: w311 -> [_ w382 _]
              tunnel: w344 -> [_ w381 _]
              tunnel: "downfactor" -> [_ w380 _]
              tunnel: [_ w379 _] -> w320
              tunnel: [_ w378 _] -> w319
              tunnel: w312 -> [_ w377 _]
              frame #0 {
                n125 = call "Set Current Directory.vi"("Set Directory"=path "E:/LabviewStuff/GPU_HK/LabVIEW Example") -> ()  [unwired: 4 in, 1 out]
                n126 = Tick Count (ms)() -> (millisecond timer value=w376:u32)
              }
              frame #1 {
                n127 = disable-structure shown="Disabled" {
                  disable-tunnel: w400 -> [w425 _]
                  disable-tunnel: w399 -> [w424 _]
                  disable-tunnel: w398 -> [w423 _]
                  disable-tunnel: w397 -> [w422 _]
                  disable-tunnel: w396 -> [w421 _]
                  disable-tunnel: w395 -> [w420 _]
                  disable-tunnel: w394 -> [w419 _]
                  disable-tunnel: w393 -> [w418 _]
                  disable-tunnel: w392 -> [w417 _]
                  disable-tunnel: w391 -> [w416 _]
                  disable-tunnel: w390 -> [w415 _]
                  disable-tunnel: w389 -> [w413 _]
                  disable-tunnel: [w412 _] -> w388
                  disable-tunnel: [w411 _] -> w387
                  disable-tunnel: [w410 _] -> w386
                  disable-tunnel: w385 -> [w409 _]
                  disable-tunnel: w384 -> [w408 _]
                  disable-tunnel: w383 -> [w407 _]
                  disable-tunnel: w382 -> [w406 _]
                  disable-tunnel: w381 -> [w405 _]
                  disable-tunnel: w380 -> [w404 _]
                  disable-tunnel: [w403 _] -> w379
                  disable-tunnel: [w402 _] -> w378
                  disable-tunnel: w377 -> [w401 _]
                  frame Disabled {
                    # "RF image log comprssed\nby GPU and scaled"
                    n128 = dll-call lib="D:/LabVIEWSuite_64_OS/GPU_HK/LabVIEW Example/riversideSAFilter-X64.dll" fn="SAbeamformerFilter"("RF_Out"=w415, "RFimage"=w415, "RFdata"=w425, "numScanline"=w424, "dataVectorLength"=w423, "TdrGeometry"=w422, "numChannel"=w421, "txPos"=w408, "rxPos"=w407, "numTxRxPair"=w420, "weighting"=w419, "fs"=w418, "sos"=w417, "time_start"=w416, "BPfilter"=w413, "DataFlag"=0, "filter"=w409, "BPFILTERLENGTH"=w405, "FILTERLENGTH"=w406, "downfactor"=w404, "Adbits"=w401) -> ("nError"=w412:i32, "RF_Out"=w411:i16[], "RFimage"=w410:i16[], "numScanline"=w402:i32, "dataVectorLength"=w403:i32)  [unwired: 20 in, 2 out]
                  }
                  frame Enabled {
                  }
                }
              }
              frame #2 {
                n129 = call "Set Current Directory.vi"("Set Directory"=w426) -> ()  [unwired: 4 in, 1 out]
                n130 = Tick Count (ms)() -> (millisecond timer value=w427:u32)
              }
            }
            "nError" <- w369
            n131 = Subtract(x=w361, y=w360) -> (x-y=→"GPU time (ms)":u32)
            n132 = Reshape Array(w363, w319, w320) -> (w310:i16[][])
            n133 = Reshape Array(w321, w319, w320) -> (w309:i16[][])
          }
          frame 2 {
            n134 = Unbundle By Name(w487) -> ("A/D info.# rf points per line"=w510:u16, "A/D info.sample rate MHz"=w497:u16, "A/D info.# lines per scan"=w509:u16, "A/D info.# A/D bits"=w477:i16)
            n135 = Reshape Array(w493, 4 ("dimension size"), 5 ("dimension size")) -> (w490:string[][])
            n136 = Transpose 2D Array(2D array=w490) -> (transposed array=w489:string[][])
            n137 = Multiply(x=1000000.0, y=w497) -> (x*y=w511:dbl)
            n138 = for {
              N: w514 -> [_]
              tunnel: w499 -> [w629]
              tunnel: w508 -> [w628]
              tunnel: w510 -> [w627]
              tunnel: w511 -> [w626]
              tunnel: w520 -> [w625]
              tunnel: w496 -> [w624]
              tunnel: w505 -> [w623]
              tunnel: w519 -> [w622]
              tunnel: [w621] -> w517 mode=indexing
              tunnel: [w620] -> w516 mode=indexing
              tunnel: w515 -> [w619]
              tunnel: [w617] -> w513 mode=indexing
              tunnel: [w616] -> w512 mode=indexing
              tunnel: w486 -> [w615]
              i -> [w618]
              n139 = call "CalcFZones.vi"("F- zones"=w628, "# rf points per line"=w627, "Radii (m)"=w619, "ROC (m)"=w625, "Sampling Rate"=w626, "delay (mm)"=w629, "# Elements"=w615, "c (m/s)"=w624, "Round to ROC?"=w623, "File index number"=w618, "One Way Receive"=w622) -> ("ZoneStart"=w621:sgl[], "ZoneShift"=w620:sgl[], "ZoneLength"=w616:sgl[], "IndexVals"=w617:sgl[])  [unwired: 3 in, 2 out]
            }
            n140 = Initialize Array(0.0, w509, w510) -> (w479:dbl[][])
            n141 = New Data Value Reference(data value=w479) -> (data value reference=w478:refnum<data-value>)  [unwired: 1 in, 1 out]
            n142 = for {
              tunnel: w495 -> [w531]
              tunnel: w478 -> [w532]
              tunnel: [w525] -> w503 mode=indexing
              tunnel: w501 -> [w530]
              tunnel: w498 -> [w529]
              tunnel: w497 -> [w528]
              tunnel: w489 -> [w527] mode=indexing
              tunnel: w494 -> [w526]
              tunnel: w477 -> [w523]
              n143 = for {
                tunnel: w531 -> [w544]
                tunnel: w530 -> [w535]
                tunnel: w529 -> [w534]
                tunnel: w528 -> [w536]
                tunnel: w527 -> [w543] mode=indexing
                tunnel: w526 -> [w542]
                tunnel: w532 -> [w540]
                tunnel: [w539] -> w524
                tunnel: w523 -> [w533]
                n144 = Concatenate Strings(w542, w543) -> (w545:string)
                n145 = Build Path(base path=w544, name or relative path=w545) -> (appended path=w541:path)
                n146 = call <vilib>:"Check if File or Folder Exists.vi"("path"=w541) -> ("file or folder exists?"=w538:bool)  [unwired: 8 in, 2 out]
                n147 = call "ReadEyeFileFast.vi"("new file path"=w541) -> ("2-D data array"=w537:sgl[][])  [unwired: 1 in, 17 out]
                n148 = call-poly "FastArraySumPoly.vi"("2-D data array"=w537, "sample rate MHz"=w536, "Type of Mean"=w535, "Bit Depth"=w533, "Perform Sum?"=w538, "Filter Prams"=w534, "Data Value Reference in"=w540) -> ("Data Value Reference out"=w539:refnum<data-value>)  [unwired: 4 in]
              }
              n149 = Delete Data Value Reference(data value reference=w524) -> (data value=w525:dbl[][])  [unwired: 1 in, 1 out]
            }
            n150 = New Data Value Reference(data value=w479) -> (data value reference=w484:refnum<data-value>)  [unwired: 1 in, 1 out]
            n151 = New Data Value Reference(data value=w479) -> (data value reference=w485:refnum<data-value>)  [unwired: 1 in, 1 out]
            n152 = Divide(x=w503, y=4) -> (x/y=w502:dbl[][][])
            n153 = for {
              tunnel: w477 -> [w565]
              tunnel: w498 -> [w554]
              tunnel: w518 -> [w568] mode=indexing
              tunnel: w501 -> [w567]
              tunnel: w504 -> [w553] mode=indexing
              tunnel: w517 -> [w566] mode=indexing
              tunnel: w516 -> [w558] mode=indexing
              tunnel: w506 -> [w564]
              tunnel: w513 -> [w563] mode=indexing
              tunnel: w512 -> [w562] mode=indexing
              tunnel: w502 -> [w556]
              tunnel: w500 -> [w555]
              tunnel: w493 -> [w551] mode=indexing
              tunnel: w495 -> [w550]
              tunnel: w494 -> [w549]
              tunnel: [w546] -> w488 mode=indexing
              tunnel: w485 -> [w560]
              tunnel: [w569] -> w482
              tunnel: w484 -> [w559]
              tunnel: [w561] -> w481
              i -> [w557]
              n154 = Concatenate Strings(w549, w551) -> (w552:string)
              n155 = Build Path(base path=w550, name or relative path=w552) -> (appended path=w548:path)
              n156 = call <vilib>:"Check if File or Folder Exists.vi"("path"=w548) -> ("file or folder exists?"=w547:bool)  [unwired: 8 in, 2 out]
              n157 = case shown="True" w547 {
                tunnel: [w571 w576] -> w569
                tunnel: w568 -> [_ w607]
                tunnel: w567 -> [_ w606]
                tunnel: w566 -> [_ w605]
                tunnel: w565 -> [_ w572]
                tunnel: w564 -> [_ w603]
                tunnel: w563 -> [_ w602]
                tunnel: w562 -> [_ w601]
                tunnel: [w570 w574] -> w561
                tunnel: w560 -> [w571 w577]
                tunnel: w559 -> [w570 w575]
                tunnel: w558 -> [_ w600]
                tunnel: w557 -> [_ w599]
                tunnel: w556 -> [_ w597]
                tunnel: w555 -> [_ w583]
                tunnel: w554 -> [_ w593]
                tunnel: w553 -> [_ w588]
                tunnel: w548 -> [_ w592]
                tunnel: [_ w589] -> w546
                frame False {
                }
                frame True {
                  # "Took out voltage scaling"
                  n158 = call "ReadEyeFileFast.vi"("new file path"=w592) -> ("RF Att"=w586:sgl, "2-D data array"=w595:sgl[][], "Header In"=w585:T7)  [unwired: 1 in, 15 out]
                  n159 = Quotient & Remainder(x=w599, y=5) -> (x-y*floor(x/y)=w596:i32)  [unwired: 1 out]
                  n160 = Add(x=w586, y=w607) -> (x+y=w604:sgl)
                  n161 = Unbundle By Name(w585) -> ("A/D info.sample rate MHz"=w587:u16)
                  n162 = Index Array(array=w597, index (dim 0)=w596) -> (element=w594:dbl[][])  [unwired: 2 in]
                  n163 = Strip Path(path=w592) -> (stripped path=w579:path, name=w582:string)
                  n164 = call "SubMean.vi"("Bit Depth"=w572, "Scan Data In"=w595, "Samp Rate (MHz)"=w587, "Filter Prams"=w593, "Type of Mean"=w606) -> ("Array"=w591:dbl[][])  [unwired: 1 in, 2 out]
                  n165 = case shown="0, Default" w588 {
                    selector: w588 -> [w608 _]
                    tunnel: w591 -> [w612 w614]
                    tunnel: [w611 w614] -> w590
                    tunnel: [w609 i16 1] -> w589
                    frame 0, Default {
                      n166 = Not Equal To 0?(x=w608) -> (x != 0?=w610:bool)
                      n167 = Multiply(x=w612, y=w608) -> (x*y=w611:dbl[][])
                      n168 = Boolean To (0,1)(Boolean=w610) -> (0, 1=w609:i16)
                    }
                    frame 1 {
                    }
                  }
                  n169 = Concatenate Strings("S", w582) -> (w580:string)
                  n170 = Subtract(x=w594, y=w590) -> (x-y=w573:dbl[][])
                  n171 = call "TimeShiftFocii.vi"("Array data"=w573, "ZoneStart"=w605, "ZoneShift"=w600, "ZoneLength"=w601, "IndexVals"=w602, "attn_dB"=w604, "Scale Voltage?"=w603, "A/D info.# A/D bits"=w572) -> ("Synth App Out"=w578:dbl[][])  [unwired: 11 in]
                  n172 = Build Path(base path=w579, name or relative path=w580) -> (appended path=w584:path)
                  n173 = call-poly "FastArraySumPoly.vi"("2-D data array"=w573, "Bit Depth"=w572, "Data Value Reference in"=w575) -> ("Data Value Reference out"=w574:refnum<data-value>)  [unwired: 8 in]
                  n174 = call-poly "FastArraySumPoly.vi"("2-D data array"=w578, "Bit Depth"=w572, "Data Value Reference in"=w577) -> ("Data Value Reference out"=w576:refnum<data-value>)  [unwired: 8 in]
                  n175 = call "SaveDataFast.vi"("Header In"=w585, "Save?"=w583, "Data Array"=w573, "File Name and Path"=w584) -> ()  [unwired: 7 in, 1 out]
                }
              }
            }
            n176 = Delete Data Value Reference(data value reference=w482) -> (data value=w483:dbl[][])  [unwired: 1 in, 1 out]
            n177 = Delete Data Value Reference(data value reference=w481) -> (data value=w480:dbl[][])  [unwired: 1 in, 1 out]
          }
          frame 3 {
            n178 = Build Array(w652) -> (w645:path[])
            n179 = Unbundle By Name(w644) -> ("A/D info.# rf points per line"=w658:u16, "A/D info.sample rate MHz"=w647:u16, "A/D info.# lines per scan"=w657:u16, "A/D info.# A/D bits"=w630:i16)
            n180 = for {
              tunnel: w645 -> [w679] mode=indexing
              tunnel: w650 -> [w677]
              tunnel: [w676] -> w635 mode=indexing
              tunnel: w648 -> [w675]
              tunnel: w647 -> [w674]
              tunnel: [w673] -> w632
              tunnel: [w672] -> w631 mode=indexing
              tunnel: w630 -> [w671]
              n181 = call "ReadEyeFileFast.vi"("new file path"=w679) -> ("RF Att"=w672:sgl, "2-D data array"=w678:sgl[][], "Header In"=w673:T7)  [unwired: 1 in, 15 out]
              n182 = call "SubMean.vi"("Bit Depth"=w671, "Scan Data In"=w678, "Samp Rate (MHz)"=w674, "Filter Prams"=w675, "Type of Mean"=w677) -> ("Array"=w676:dbl[][])  [unwired: 1 in, 2 out]
            }
            n183 = Multiply(x=1000000.0, y=w647) -> (x*y=w659:dbl)
            n184 = for {
              N: w662 -> [_]
              tunnel: w649 -> [w736]
              tunnel: w656 -> [w735]
              tunnel: w658 -> [w734]
              tunnel: w659 -> [w733]
              tunnel: w668 -> [w732]
              tunnel: w646 -> [w731]
              tunnel: w654 -> [w730]
              tunnel: w667 -> [w729]
              tunnel: [w728] -> w665 mode=indexing
              tunnel: [w727] -> w664 mode=indexing
              tunnel: w663 -> [w726]
              tunnel: [w724] -> w661 mode=indexing
              tunnel: [w723] -> w660 mode=indexing
              tunnel: w643 -> [w722]
              i -> [w725]
              n185 = call "CalcFZones.vi"("F- zones"=w735, "# rf points per line"=w734, "Radii (m)"=w726, "ROC (m)"=w732, "Sampling Rate"=w733, "delay (mm)"=w736, "# Elements"=w722, "c (m/s)"=w731, "Round to ROC?"=w730, "File index number"=w725, "One Way Receive"=w729) -> ("ZoneStart"=w728:sgl[], "ZoneShift"=w727:sgl[], "ZoneLength"=w723:sgl[], "IndexVals"=w724:sgl[])  [unwired: 3 in, 2 out]
            }
            n186 = Initialize Array(0.0, w657, w658) -> (w642:dbl[][])
            n187 = New Data Value Reference(data value=w642) -> (data value reference=w640:refnum<data-value>)  [unwired: 1 in, 1 out]
            n188 = New Data Value Reference(data value=w642) -> (data value reference=w641:refnum<data-value>)  [unwired: 1 in, 1 out]
            n189 = Bundle By Name(cluster=w632, "A/D info.# A/D bits"=i16 8) -> (w633:T7)
            n190 = for {
              tunnel: w645 -> [w699] mode=indexing
              tunnel: w630 -> [w711]
              tunnel: w648 -> [_]
              tunnel: w666 -> [w713] mode=indexing
              tunnel: w650 -> [_]
              tunnel: w653 -> [w696] mode=indexing
              tunnel: w665 -> [w712] mode=indexing
              tunnel: w664 -> [w706] mode=indexing
              tunnel: w655 -> [w709]
              tunnel: w661 -> [w708] mode=indexing
              tunnel: w660 -> [w707] mode=indexing
              tunnel: w635 -> [w700]
              tunnel: w642 -> [w697]
              tunnel: w651 -> [w684]
              tunnel: w641 -> [w692]
              tunnel: [w694] -> w638
              tunnel: w640 -> [w693]
              tunnel: [w695] -> w639
              tunnel: w635 -> [w683] mode=indexing
              tunnel: w633 -> [w682]
              tunnel: w631 -> [w681] mode=indexing
              tunnel: w630 -> [w680]
              i -> [w703]
              w702 = 5
              # "Took out voltage scaling"
              n191 = Quotient & Remainder(x=w703, y=w702) -> (floor(x/y)=w705:i32)  [unwired: 1 out]
              n192 = Subtract(x=w703, y=w702) -> (x-y=w701:i32)
              n193 = case shown="1, Default" w705 {
                tunnel: w701 -> [_ w717]
                tunnel: w700 -> [_ w716]
                tunnel: [w714 w715] -> w698
                tunnel: w697 -> [w714 _]
                frame 0 {
                }
                frame 1, Default {
                  n194 = Index Array(array=w716, index (dim 0)=w717) -> (element=w715:dbl[][])  [unwired: 2 in]
                }
              }
              n195 = Add(x=w681, y=w713) -> (x+y=w710:sgl)
              n196 = case shown="0, Default" w696 {
                selector: w696 -> [w718 _]
                tunnel: w683 -> [w720 w721]
                tunnel: [w719 w721] -> w704
                frame 0, Default {
                  n197 = Multiply(x=w720, y=w718) -> (x*y=w719:dbl[][])
                }
                frame 1 {
                }
              }
              n198 = Strip Path(path=w699) -> (stripped path=w687:path, name=w690:string)
              n199 = Concatenate Strings("S", w690) -> (w688:string)
              n200 = Subtract(x=w704, y=w698) -> (x-y=w685:dbl[][])
              n201 = call "TimeShiftFocii.vi"("Array data"=w685, "ZoneStart"=w712, "ZoneShift"=w706, "ZoneLength"=w707, "IndexVals"=w708, "attn_dB"=w710, "Scale Voltage?"=w709, "A/D info.# A/D bits"=w711) -> ("Synth App Out"=w691:dbl[][])  [unwired: 11 in]
              n202 = Build Path(base path=w687, name or relative path=w688) -> (appended path=w686:path)
              n203 = call-poly "FastArraySumPoly.vi"("2-D data array"=w691, "Bit Depth"=w680, "Data Value Reference in"=w692) -> ("Data Value Reference out"=w694:refnum<data-value>)  [unwired: 8 in]
              n204 = call-poly "FastArraySumPoly.vi"("2-D data array"=w685, "Bit Depth"=w680, "Data Value Reference in"=w693) -> ("Data Value Reference out"=w695:refnum<data-value>)  [unwired: 8 in]
              n205 = call "SaveDataFast.vi"("Header In"=w682, "Save?"=w684, "Data Array"=w685, "File Name and Path"=w686) -> ()  [unwired: 7 in, 1 out]
            }
            n206 = Delete Data Value Reference(data value reference=w638) -> (data value=w637:dbl[][])  [unwired: 1 in, 1 out]
            n207 = Delete Data Value Reference(data value reference=w639) -> (data value=w636:dbl[][])  [unwired: 1 in, 1 out]
          }
          frame 4 {
            n208 = Unbundle By Name(w743) -> ("A/D info.# rf points per line"=w761:u16, "A/D info.sample rate MHz"=w762:u16, "A/D info.# lines per scan"=w760:u16, "A/D info.# A/D bits"=w769:i16, "Comment"=w737:string)
            n209 = local write "Comment"(w737) -> ()
            n210 = call "CalcPixelShifts.vi"("Sampling Rate (Hz)"=w762, "c (m/s)"=w748, "delay (mm)"=w750, "rf pts"=w761, "ROC (m)"=w768, "Radii (m)"=w763, "One Way Receive"=w764, "Dual mode"=w739) -> ("InterpIndex"=w741:sgl[][])  [unwired: 7 in]
            n211 = Initialize Array(0.0, w760, w761) -> (w754:dbl[][])
            n212 = New Data Value Reference(data value=w754) -> (data value reference=w753:refnum<data-value>)  [unwired: 1 in, 1 out]
            n213 = New Data Value Reference(data value=w754) -> (data value reference=w757:refnum<data-value>)  [unwired: 1 in, 1 out]
            n214 = for {
              tunnel: w769 -> [w789]
              tunnel: w766 -> [w791]
              tunnel: w767 -> [w792]
              tunnel: w759 -> [w782]
              tunnel: w765 -> [w790]
              tunnel: w740 -> [w780] mode=indexing
              tunnel: w758 -> [w788]
              tunnel: w741 -> [w787] mode=indexing
              tunnel: w757 -> [w786]
              tunnel: [w785] -> w756
              tunnel: w753 -> [w784]
              tunnel: [w783] -> w752
              tunnel: [w781] -> w749 mode=indexing
              tunnel: w747 -> [w779]
              tunnel: w746 -> [w778]
              tunnel: w745 -> [w776]
              tunnel: w744 -> [w775] mode=indexing
              tunnel: w738 -> [w771]
              workers-P: _ -> [_]
              n215 = Concatenate Strings(w776, w775) -> (w774:string)
              n216 = Build Path(base path=w778, name or relative path=w774) -> (appended path=w772:path)
              n217 = call <vilib>:"Check if File or Folder Exists.vi"("path"=w772) -> ("file or folder exists?"=w773:bool, "dup path"=w777:path)  [unwired: 8 in, 1 out]
              n218 = case shown="True" w773 {
                tunnel: w792 -> [_ w817]
                tunnel: w791 -> [_ w816]
                tunnel: w777 -> [_ w815]
                tunnel: w790 -> [_ w802]
                tunnel: w789 -> [_ w805]
                tunnel: w788 -> [_ _]
                tunnel: w787 -> [_ w795]
                tunnel: w786 -> [w794 w811]
                tunnel: [w794 w810] -> w785
                tunnel: w784 -> [w793 w809]
                tunnel: [w793 w808] -> w783
                tunnel: w782 -> [_ w804]
                tunnel: [_ w813] -> w781
                tunnel: w780 -> [_ w812]
                tunnel: w779 -> [_ _]
                tunnel: w771 -> [_ w798]
                frame False {
                }
                frame True {
                  w807 = TRUE ("Perform Sum?")
                  n219 = call "ReadEyeFileFast.vi"("new file path"=w815) -> ("2-D data array"=w800:sgl[][], "Header In"=w801:T7)  [unwired: 1 in, 16 out]
                  n220 = Array Subset(array=w800, index (col)=w798) -> (w799:sgl[][])  [unwired: 3 in]
                  n221 = Unbundle By Name(w801) -> ("A/D info.sample rate MHz"=w803:u16)
                  n222 = call "SubMean.vi"("Bit Depth"=w805, "Scan Data In"=w799, "Samp Rate (MHz)"=w803, "Filter Prams"=w804, "Type of Mean"=w802) -> ("Array"=w806:dbl[][])  [unwired: 1 in, 2 out]
                  n223 = case shown="True" w817 {
                    tunnel: [w825 w828] -> w814
                    tunnel: w806 -> [w825 w827]
                    tunnel: w816 -> [_ w826]
                    frame False {
                    }
                    frame True {
                      n224 = call "Compress Chirp.vi"("Chirp"=w826, "Array In"=w827) -> ("Array Out"=w828:dbl[][])
                    }
                  }
                  n225 = case shown="0" w812 {
                    selector: w812 -> [w818 _]
                    tunnel: w814 -> [w822 w824]
                    tunnel: [w821 w824] -> w797
                    tunnel: [w819 i16 1] -> w813
                    frame 0 {
                      n226 = Not Equal To 0?(x=w818) -> (x != 0?=w820:bool)
                      n227 = Multiply(x=w822, y=w818) -> (x*y=w821:dbl[][])
                      n228 = Boolean To (0,1)(Boolean=w820) -> (0, 1=w819:i16)
                    }
                    frame 1, Default {
                    }
                  }
                  n229 = call "PixelInterp.vi"("IndexVals"=w795, "Array data"=w797) -> ("Synth App Out"=w796:dbl[][])  [unwired: 6 in]
                  n230 = call-poly "FastArraySumPoly.vi"("2-D data array"=w796, "sample rate MHz"=w803, "Type of Mean"=w802, "Bit Depth"=w805, "Perform Sum?"=w807, "Filter Prams"=w804, "Data Value Reference in"=w811) -> ("Data Value Reference out"=w810:refnum<data-value>)  [unwired: 4 in]
                  n231 = call-poly "FastArraySumPoly.vi"("2-D data array"=w797, "sample rate MHz"=w803, "Type of Mean"=w802, "Bit Depth"=w805, "Perform Sum?"=w807, "Filter Prams"=w804, "Data Value Reference in"=w809) -> ("Data Value Reference out"=w808:refnum<data-value>)  [unwired: 4 in]
                }
              }
            }
            n232 = Delete Data Value Reference(data value reference=w752) -> (data value=w751:dbl[][])  [unwired: 1 in, 1 out]
            n233 = Delete Data Value Reference(data value reference=w756) -> (data value=w755:dbl[][])  [unwired: 1 in, 1 out]
          }
        }
      }
      frame #3 {
        w843 = 0.1
        # "Rescale to n bits"
        n234 = Unbundle By Name(w840) -> ("A/D info.# A/D bits"=w839:i16)
        n235 = Decrement(x=w839) -> (x-1=w838:i16)
        n236 = Add Array Elements(numeric array=w841) -> (sum=w836:i32)
        n237 = Power Of 2(x=w838) -> (2^x=w837:dbl)
        n238 = Multiply(x=w837, y=w836) -> (x*y=w835:dbl)
        n239 = Subtract(x=w835, y=2) -> (x-y=w846:dbl)
        n240 = for {
          N: w846 -> [_]
          tunnel: [w862] -> w848 mode=indexing
          i -> [w863]
          n241 = case shown="1, Default" w863 {
            selector: w863 -> [_ w865]
            tunnel: [1 w865] -> w862
            frame 0 {
            }
            frame 1, Default {
            }
          }
        }
        n242 = Array Max & Min(array=w834) -> (max value=w855:dbl, min value=w859:dbl)  [unwired: 2 out]
        n243 = Array Max & Min(array=w833) -> (max value=w856:dbl, min value=w858:dbl)  [unwired: 2 out]
        n244 = Absolute Value(x=w859) -> (abs(x)=w854:dbl)
        n245 = Absolute Value(x=w858) -> (abs(x)=w857:dbl)
        n246 = Index Array(array=w834, index (row)="index (row)") -> (element=w832:dbl[])  [unwired: 1 in]
        n247 = Max & Min(x=w855, y=w854) -> (max(x,y)=w853:dbl)  [unwired: 1 out]
        n248 = Max & Min(x=w856, y=w857) -> (max(x,y)=w852:dbl)  [unwired: 1 out]
        n249 = Max & Min(x=w853, y=w852) -> (max(x,y)=w860:dbl)  [unwired: 1 out]
        n250 = Divide(x=w848, y=w835) -> (x/y=w847:dbl[])
        n251 = expression code="20*log(x)"(w847) -> (w844:dbl[])
        n252 = expression code="20*log(2*x)"(w860) -> (w861:dbl)
        n253 = Index Array(array=w833, index (row)="index (row)") -> (element=w829:dbl[])  [unwired: 1 in]
        n254 = Build Array(w832, w829) -> (→"Waveform Graph":dbl[][])
        n255 = Build Array (concatenate)(w844, w843, w843) -> (w842:dbl[])
        n256 = case shown="True" w851 {
          tunnel: w834 -> [_ w872]
          tunnel: w833 -> [_ w873]
          tunnel: w849 -> [_ w870]
          tunnel: w842 -> [_ w867]
          frame False {
          }
          frame True {
            n257 = Transpose 2D Array(2D array=w872) -> (transposed array=w871:dbl[][])
            n258 = Transpose 2D Array(2D array=w873) -> (transposed array=w869:dbl[][])
            n259 = case shown="0, Default" w870 {
              tunnel: w871 -> [w878 w895 w898]
              tunnel: [w875 w894 w897] -> w866
              tunnel: w869 -> [w877 w892 _]
              tunnel: [w874 w891 _] -> w868
              tunnel: w867 -> [w876 _ _]
              frame 0, Default {
                n260 = for {
                  tunnel: w878 -> [w883] mode=indexing
                  tunnel: w877 -> [w882] mode=indexing
                  tunnel: w876 -> [w881]
                  tunnel: [w880] -> w875 mode=indexing
                  tunnel: [w879] -> w874 mode=indexing
                  n261 = for {
                    tunnel: w883 -> [w890] mode=indexing
                    tunnel: w882 -> [w889] mode=indexing
                    tunnel: w881 -> [w888]
                    tunnel: [w887] -> w880 mode=indexing
                    tunnel: [w886] -> w879 mode=indexing
                    n262 = Absolute Value(x=w889) -> (abs(x)=w884:dbl)
                    n263 = Absolute Value(x=w890) -> (abs(x)=w885:dbl)
                    n264 = Index Array(array=w888, index=w885) -> (element=w887:dbl)
                    n265 = Index Array(array=w888, index=w884) -> (element=w886:dbl)
                  }
                }
              }
              frame 22 {
                n266 = call <vilib>:"Quick Scale 2D.vi"("X"=w895) -> ("Yij=Xij/Max|X|"=w896:dbl[][])  [unwired: 2 out]
                n267 = call <vilib>:"Quick Scale 2D.vi"("X"=w892) -> ("Yij=Xij/Max|X|"=w893:dbl[][])  [unwired: 2 out]
                n268 = expression code="20*log(abs(x))"(w896) -> (w894:dbl[][])
                n269 = expression code="20*log(abs(x))"(w893) -> (w891:dbl[][])
              }
              frame 11 {
                n270 = Array Max & Min(array=w898) -> (max value=w899:dbl)  [unwired: 3 out]
                n271 = Subtract(x=w898, y=w899) -> (x-y=w897:dbl[][])
              }
            }
            "Synth Aperture" <- w866
            "Raw Summation" <- w868
          }
        }
        n272 = Tick Count (ms)() -> (millisecond timer value=w850:u32)
      }
      frame #4 {
        n273 = case shown="True" w906 {
          tunnel: w907 -> [_ w921]
          tunnel: w905 -> [_ w916]
          tunnel: w904 -> [_ w913]
          tunnel: w903 -> [_ w912]
          tunnel: w902 -> [_ w911]
          tunnel: w901 -> [_ w910]
          tunnel: w900 -> [_ w909]
          frame False {
          }
          frame True {
            n274 = Unbundle By Name(w921) -> ("A/D info.sample rate MHz"=w917:u16)
            n275 = Reciprocal(x=w917) -> (1/x=w923:dbl)
            n276 = case shown="True" w916 {
              tunnel: [2000 1000] -> w915
              tunnel: w910 -> [w924 w927]
              tunnel: [w924 w926] -> w914
              frame False {
              }
              frame True {
                n277 = expression code="2*x"(w927) -> (w926:dbl)
              }
            }
            n278 = Divide(x=w909, y=w915) -> (x/y=w922:dbl)
            n279 = case shown="True" "Axis scaling" {
              tunnel: [w930 w936] -> w918
              tunnel: w923 -> [_ w942]
              tunnel: w921 -> [_ w941]
              tunnel: [w930 w937] -> w919
              tunnel: [0 w931] -> w908
              tunnel: w922 -> [_ w938]
              tunnel: w914 -> [_ w932]
              tunnel: w913 -> [_ w935]
              tunnel: w912 -> [_ w934]
              tunnel: w911 -> [_ w933]
              frame False {
                w930 = 1
              }
              frame True {
                n280 = case shown="1" w935 {
                  tunnel: w934 -> [_ w944]
                  tunnel: w933 -> [_ w949]
                  tunnel: w932 -> [w943 w948]
                  tunnel: [w943 w947] -> w931
                  frame 0, Default {
                  }
                  frame 1 {
                    n281 = Index Array(array=w949, index=9) -> (element=w945:dbl)
                    n282 = formula code="d=1000*(R-(R**2-a**2)**0.5);\nd=0;"("R"=w944, "a"=w945) -> ("d"=w946:dbl)
                    n283 = Add(x=w948, y=w946) -> (x+y=w947:dbl)
                  }
                }
                n284 = Unbundle By Name(w941) -> ("Scan Settings.Distance between\nscan lines (um)"=w940:u16)
                n285 = Multiply(x=w942, y=w938) -> (x*y=w936:dbl)
                n286 = Divide(x=w940, y=1000) -> (x/y=w937:dbl)
              }
            }
            n287 = property on="Raw Summation" class="IntGraph (strict)"("X Scale.Offset and Multiplier:Multiplier"=w918, "X Scale.Offset and Multiplier:Offset"=w908, "Y Scale.Offset and Multiplier:Multiplier"=w919) -> ()  [unwired: 2 in, 2 out]
            n288 = property on="Synth Aperture" class="IntGraph (strict)"("X Scale.Offset and Multiplier:Offset"=w908, "X Scale.Offset and Multiplier:Multiplier"=w918, "Y Scale.Offset and Multiplier:Multiplier"=w919) -> ()  [unwired: 2 in, 2 out]
          }
        }
      }
      frame #5 {
        # "Create Processed Folder if saving data."
        n289 = case shown="True" w953 {
          tunnel: w951 -> [_ w957]
          tunnel: w952 -> [_ w954]
          frame False {
          }
          frame True {
            n290 = Build Path(base path=w957, name or relative path=w954) -> (appended path=w956:path)
            n291 = File/Directory Info(path=w956) -> (directory=w958:bool, error out=w955:errorcluster)  [unwired: 1 in, 5 out]
            n292 = Unbundle By Name(w955) -> ()  [unwired: 1 out]
            n293 = case shown="False" w958 {
              tunnel: w956 -> [w959 _]
              frame False {
                n294 = Create Folder(path (use dialog)=w959) -> ()  [unwired: 1 in, 4 out]
              }
              frame True {
              }
            }
          }
        }
      }
      frame #6 {
        n295 = Logarithm Base 2(1:w972) -> (0:w971:dbl)
        n296 = Increment(x=w971) -> (x+1=w969:dbl)
        n297 = Round Toward +Infinity(x=w969) -> (ceil(x): smallest int >= x=w970:dbl)
        n298 = case shown="True" w975 {
          tunnel: w980 -> [_ w984]
          tunnel: w963 -> [_ w981]
          tunnel: w962 -> [_ w1018]
          tunnel: w979 -> [_ w1012]
          tunnel: w978 -> [_ w992]
          tunnel: w967 -> [_ w986]
          tunnel: w966 -> [_ w991]
          tunnel: w977 -> [_ w1021]
          tunnel: w976 -> [_ w990]
          tunnel: w974 -> [_ w1015]
          tunnel: w973 -> [_ w1014]
          tunnel: w970 -> [_ w1013]
          tunnel: w968 -> [_ w1001]
          tunnel: w964 -> [_ w999]
          tunnel: w965 -> [_ w1007]
          tunnel: w961 -> [_ w982]
          tunnel: w960 -> [_ w983]
          frame False {
          }
          frame True {
            w988 = "Elem1" ("name or relative path")
            w987 = "Sum" ("name or relative path")
            n299 = Select(t="Norm", s=w1021, f="") -> (s? t:f=w995:string)
            n300 = Build Path(base path=w991, name or relative path=w990) -> (appended path=w989:path)
            n301 = Concatenate Strings(w995, ".eye") -> (w993:string)
            n302 = Build Path(base path=w989, name or relative path="SF") -> (appended path=w996:path)
            n303 = Concatenate Strings(w986, "SFoc", w993) -> (w1023:string)
            n304 = Concatenate Strings(w986, w987, w993) -> (w1022:string)
            n305 = Build Path(base path=w989, name or relative path=w987) -> (appended path=w997:path)
            n306 = Concatenate Strings(w986, w988, w993) -> (w1008:string)
            n307 = Build Path(base path=w989, name or relative path=w988) -> (appended path=w998:path)
            n308 = Build Path(base path=w996, name or relative path=w1023) -> (appended path=w1017:path)
            n309 = Build Path(base path=w998, name or relative path=w1008) -> (appended path=w1000:path)
            n310 = Build Path(base path=w997, name or relative path=w1022) -> (appended path=w1002:path)
            n311 = Number To Fractional String(number=w1012, precision (6)=1) -> ()  [unwired: 3 out]
            n312 = Bundle By Name(cluster=w984, "A/D info.# A/D bits"=w1013, "Misc Info.Div By or SF zones"=w992, "Patient Info.extended ID"="Syn Foc", "A/D info.# bytes per A/D"=u16 2, "Scan Info.delay"=w1015, "Misc Info.c speed"=w1014) -> (w1005:T7)
            n313 = Bundle By Name(cluster=w1005, "Patient Info.extended ID"="Sum Rings") -> (w1003:T7)
            n314 = Bundle By Name(cluster=w1005, "Patient Info.extended ID"="Center Elem") -> (w1004:T7)
            n315 = case shown="True" "Save Tiff?" {
              tunnel: w982 -> [_ w1027]
              tunnel: w989 -> [_ w1034]
              tunnel: w986 -> [_ w1032]
              tunnel: w984 -> [_ w1029]
              tunnel: w983 -> [_ w1028]
              tunnel: w981 -> [_ _]
              frame False {
              }
              frame True {
                n316 = Build Path(base path=w1034, name or relative path="TIFF") -> (appended path=w1033:path)
                n317 = Concatenate Strings(w1032, ".tif" ("name or relative path")) -> (w1030:string)
                n318 = call "HilbertLogCompress.vi"() -> ()  [unwired: 11 in, 1 out]
                n319 = call "SaveAsTiff.vi"("Data In"=w1027, "Header In"=w1029, "File Path"=w1033, "Image Name"=w1030, "pairs"=w1028) -> ()  [unwired: 7 in]
              }
            }
            n320 = call "SaveDataFast.vi"("Header In"=w1003, "Save?"=w1001, "Data Array"=w1018, "File Name and Path"=w1002) -> ()  [unwired: 7 in, 1 out]
            n321 = call "SaveDataFast.vi"("Header In"=w1004, "Save?"=w999, "Data Array"=w1007, "File Name and Path"=w1000) -> ()  [unwired: 7 in, 1 out]
            n322 = call "SaveDataFast.vi"("Header In"=w1005, "Save?"="Show SF?", "Data Array"=w981, "File Name and Path"=w1017) -> ()  [unwired: 7 in, 1 out]
          }
        }
      }
    }
    n323 = Subtract(x=w95, y=w94) -> (x-y=→"time per\nimage (ms)":u32)
  }
  n324 = for {
    N: 3 -> [_]
    tunnel: w16 -> [_]
    n325 = Wait (ms)(milliseconds to wait=u32 400) -> ()  [unwired: 1 out]
    n326 = call <vilib>:"Beep.vi"("use system alert? (T)"=FALSE, "duration (msec)"=u32 300, "frequency (Hz)"=u32 440) -> ()  [unwired: 9 in]
  }
